vi "CAEN_HVSystem.ProcCases.vi"(0 "i ref in":refnum<vi>, 1 "selector":string, 2 "Data":T1, 3 "call cluster":T2={"Object"="", "Selector"="", "CallType"=enum."synchronous", "Async Object"="", "Async Selector"="", "Data Descriptor"="", "Data"=[], "Error #"=0, "Expire"=0}, 5 "error in (no error)":errorcluster) -> (14 "i ref out":refnum<vi>, 17 "answer cluster":T2={"Object"="", "Selector"="", "CallType"=enum."synchronous", "Async Object"="", "Async Selector"="", "Data Descriptor"="", "Data"=[], "Error #"=0, "Expire"=0}, 19 "error out":errorcluster)   [LabVIEW 2014, in "CAEN_HVSystem.lvlib"]
doc: "This method is called by a process from within the default case in the event loop. The methods of a class that are linked to events will be called from THIS method. Add your code here."
uses:
  CAEN_HVSystem.lvlib
  CS_Core/CSSystem/CoreDefs/CoreDefs.call_type.ctl
  CS_Core/BaseProcess/BaseProcess.descriptor string definition.ctl
  CS_Core/CSSystem/CoreDefs/CoreDefs.rawDataType.ctl
  CS_Core/CSApplicationBaseClasses/DeviceBase/DeviceBase.deviceState.ctl
  CSlibraries/UtilityLib/UtilityLib.valueStatus.ctl
  CS_Core/CSSystem/CoreLib/CoreLib.string 2 byte array.vi
  CS_Core/CSSystem/CoreLib/CoreLib.short 2 byte array.vi
  CS_Core/CSSystem/CoreLib/CoreLib.byte array 2 string.vi
  CS_Core/CSSystem/CoreLib/CoreLib.byte array 2 short.vi
  CS_Core/CSSystem/CoreLib/CoreLib.lvlib
  CS_Core/BaseProcess/BaseProcess.lvlib
  CS_Core/CSApplicationBaseClasses/DeviceBase/DeviceBase.lvlib
  CS_Core/CAEObj/CAEObj.lvlib
  CSlibraries-extern/DimLVEvent/LVDimInterface/LVDimInterface.lvlib
  CSlibraries/UtilityLib/UtilityLib.lvlib
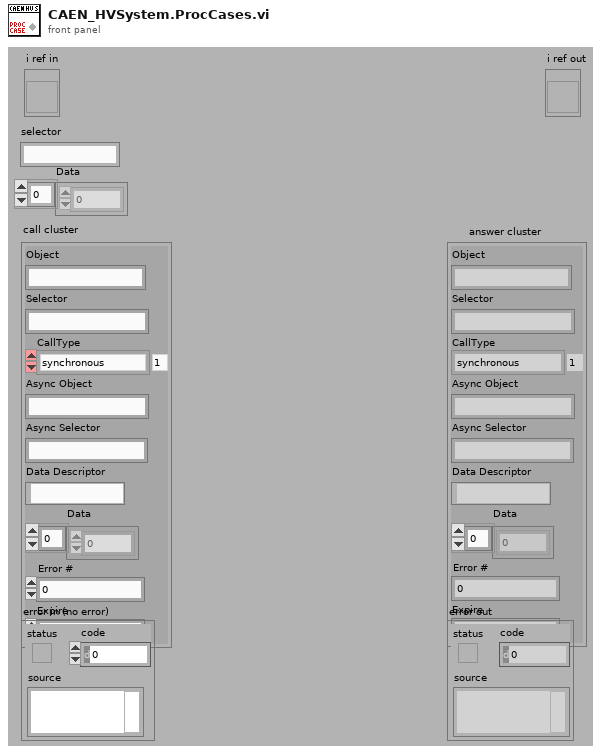
[diagram p1: front panel]
types:
  T1 = typedef "CoreDefs.rawDataType.ctl" = i8[]
  T2 = typedef "CoreDefs.call_type.ctl" = cluster{"Object":string, "Selector":string, "CallType":enum16{"simple", "synchronous", "asynchronous"}, "Async Object":string, "Async Selector":string, "Data Descriptor":T3, "Data":T1, "Error #":i32, "Expire":u32}
  T3 = typedef "BaseProcess.lvlib/BaseProcess.descriptor string definition.ctl" = string
  T4 = typedef "UtilityLib.lvlib/UtilityLib.valueStatus.ctl" = enum16{"no info available", "stand by/off", "on", "warning", "alarm/malfunction", "not implemented", "user action required", "important information", "system default", "control default", "indicator default", "button default"}
  T5 = typedef "BaseProcess.lvlib/BaseProcess.i attribute.ctl" = cluster{"EventStatus":string, "EventError":i32, "PresetEvtWatchD":i32, "PresetPdcWatchD":i32, "EventTimeout":i32, "PeriodicInterval":i32, "Interface":string[], "Address":string[], "Special":string[], "PeriodicError":i32, "PeriodicStatus":string, "SuperProc":string, "Descriptors":T6[], "CaseRef":refnum<vi>, "PdcRef":refnum<vi>, "Thread Ref":refnum<vi>, "eventErrorID":i32, "eventStatusID":i32, "periodicErrorID":i32, "periodicStatusID":i32, "pdcCtrID":i32}
  T6 = typedef "BaseProcess.lvlib/BaseProcess.descriptor definition.ctl" = cluster{"selector":string, "descriptor":T3}
  T7 = typedef "CAEN_HVSystem.lvlib/CAEN_HVSystem.i attribute.ctl" = cluster{"System Name":string, "DIM Service IDs":cluster{"Fan Status":i32}, "SymbolicName":cluster{"SymbolicName":string, "DIM Status":cluster{"no link":bool, "quality":i32, "Time Stamp":timestamp}}, "ModelName":cluster{"ModelName":string, "DIM Status":cluster{"no link":bool, "quality":i32, "Time Stamp":timestamp}}, "Slots":cluster{"Slots":i16, "DIM Status":cluster{"no link":bool, "quality":i32, "Time Stamp":timestamp}}, "Kill":cluster{"Kill":bool, "DIM Status":cluster{"no link":bool, "quality":i32, "Time Stamp":timestamp}}, "ClearAlarm":cluster{"ClearAlarm":bool, "DIM Status":cluster{"no link":bool, "quality":i32, "Time Stamp":timestamp}}, "Sessions":cluster{"Sessions":string, "DIM Status":cluster{"no link":bool, "quality":i32, "Time Stamp":timestamp}}, "SwRelease":cluster{"SwRelease":string, "DIM Status":cluster{"no link":bool, "quality":i32, "Time Stamp":timestamp}}, "GenSignCfg":cluster{"GenSignCfg":i16, "DIM Status":cluster{"no link":bool, "quality":i32, "Time Stamp":timestamp}}, "FrontPanIn":cluster{"FrontPanIn":i16, "DIM Status":cluster{"no link":bool, "quality":i32, "Time Stamp":timestamp}}, "FrontPanOut":cluster{"FrontPanOut":i16, "DIM Status":cluster{"no link":bool, "quality":i32, "Time Stamp":timestamp}}, "HvPwSM":cluster{"HvPwSM":string, "DIM Status":cluster{"no link":bool, "quality":i32, "Time Stamp":timestamp}}, "FanStat":cluster{"FanStat":string, "DIM Status":cluster{"no link":bool, "quality":i32, "Time Stamp":timestamp}}, "ClkFreq":cluster{"ClkFreq":i16, "DIM Status":cluster{"no link":bool, "quality":i32, "Time Stamp":timestamp}}, "HVClkConf":cluster{"HVClkConf":string, "DIM Status":cluster{"no link":bool, "quality":i32, "Time Stamp":timestamp}}, "CnetCrNum":cluster{"CnetCrNum":i16, "DIM Status":cluster{"no link":bool, "quality":i32, "Time Stamp":timestamp}}, "IPAddr":cluster{"IPAddr":string, "DIM Status":cluster{"no link":bool, "quality":i32, "Time Stamp":timestamp}}, "IPNetMsk":cluster{"IPNetMsk":string, "DIM Status":cluster{"no link":bool, "quality":i32, "Time Stamp":timestamp}}, "IPGw":cluster{"IPGw":string, "DIM Status":cluster{"no link":bool, "quality":i32, "Time Stamp":timestamp}}, "RS232Par":cluster{"RS232Par":string, "DIM Status":cluster{"no link":bool, "quality":i32, "Time Stamp":timestamp}}}
  T8 = typedef "DeviceBase.lvlib/DeviceBase.i attribute.ctl" = cluster{"deviceState":i32, "deviceStateID":i32, "deviceID":string, "deviceIDID":i32, "advancedGUIClass":string, "advancedGUIClassID":i32}
  T9 = typedef "DeviceBase.lvlib/DeviceBase.deviceState.ctl" = i16
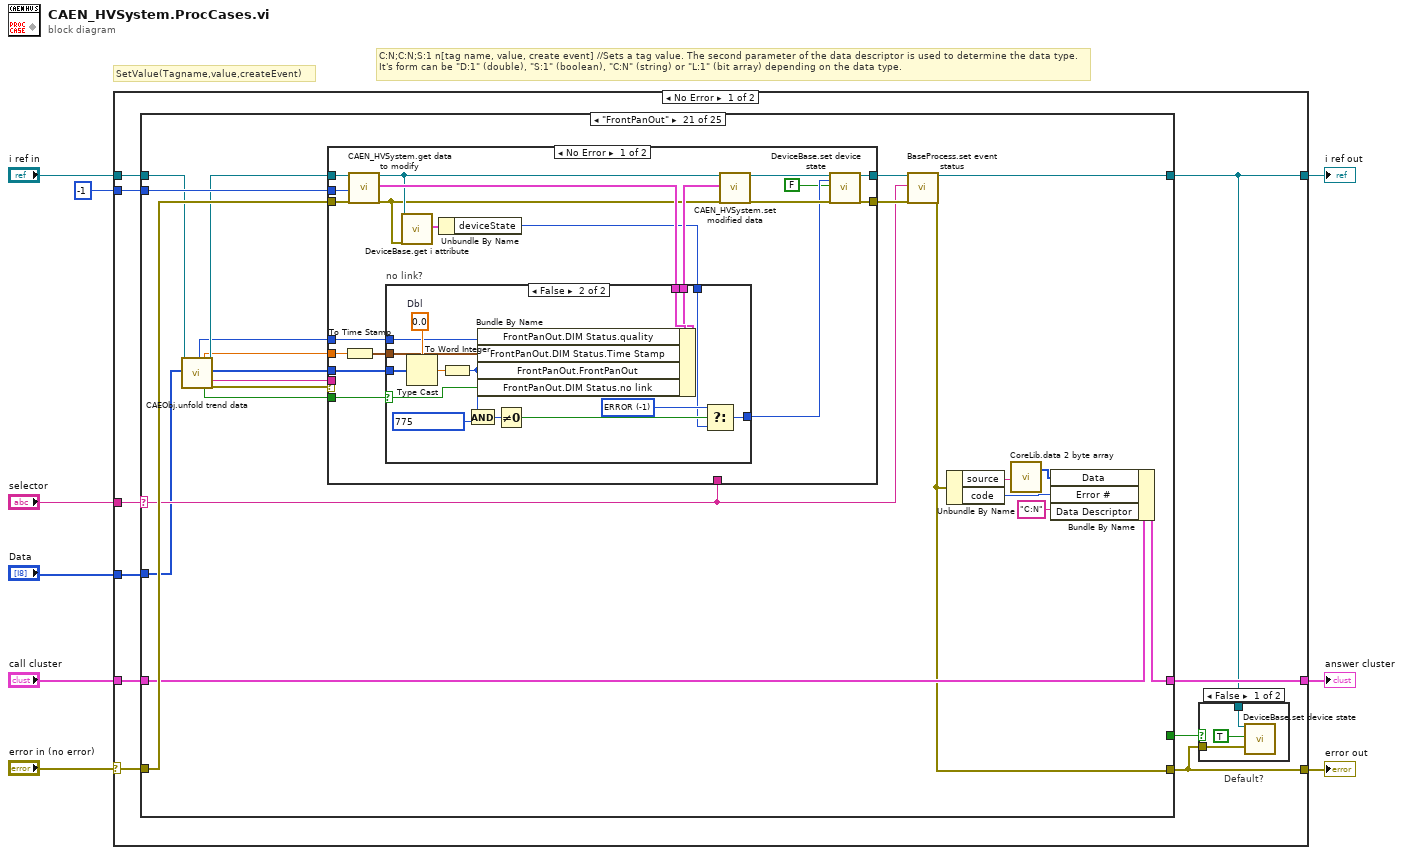
[diagram p0: block diagram]
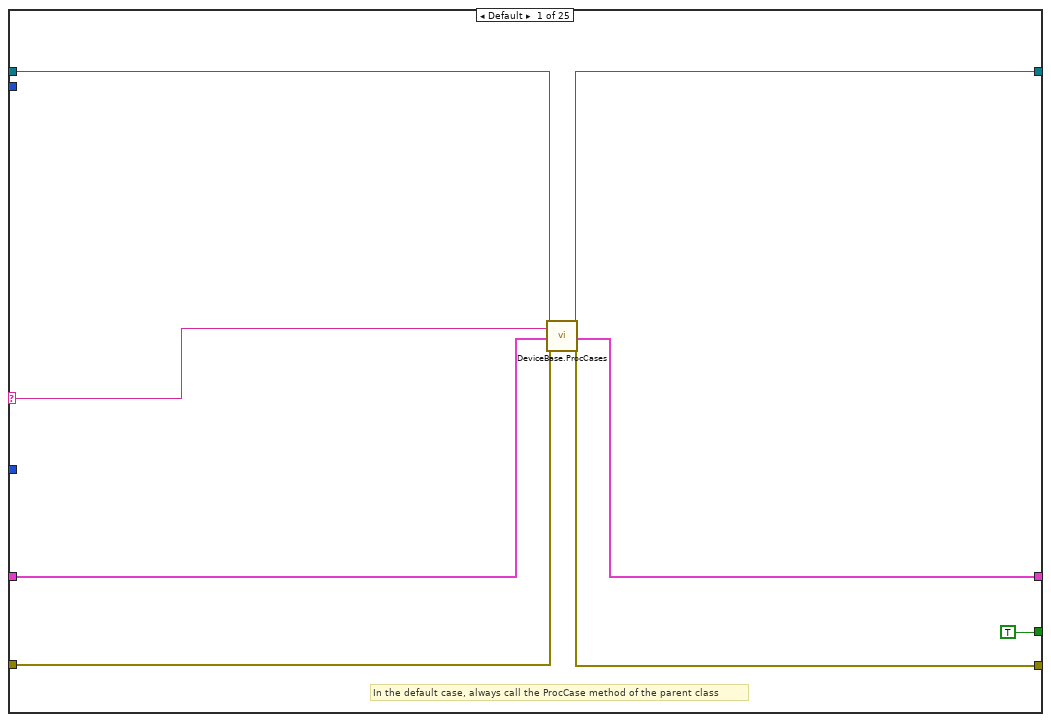
[diagram p3: hidden frame]
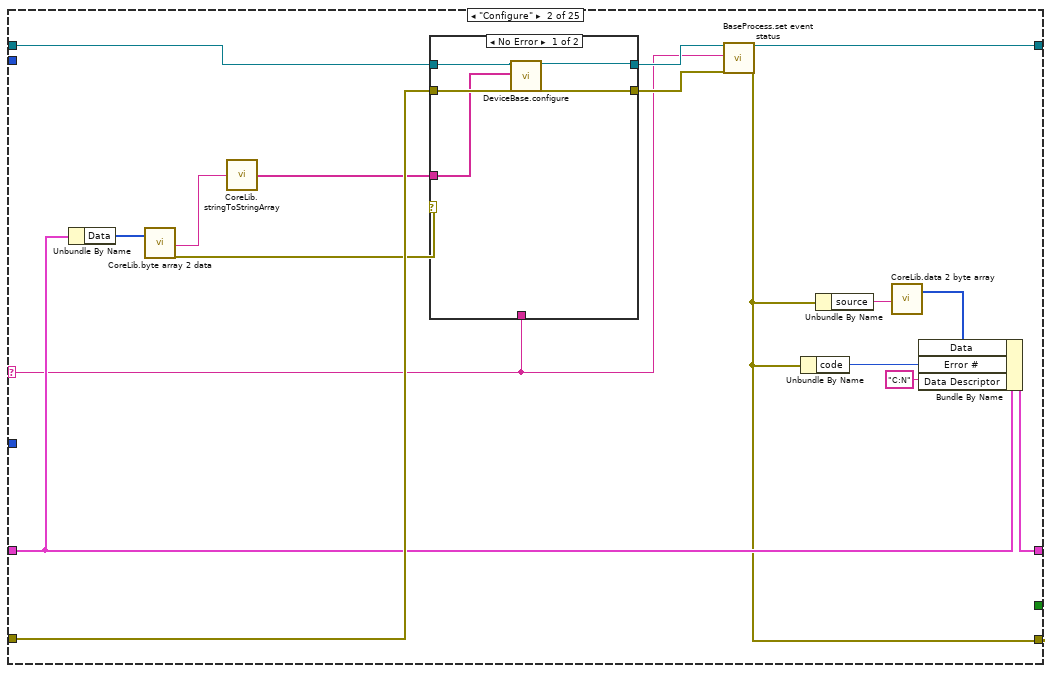
[diagram p4: hidden frame]
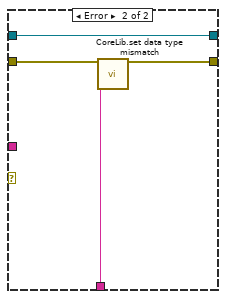
[diagram p5: hidden frame]
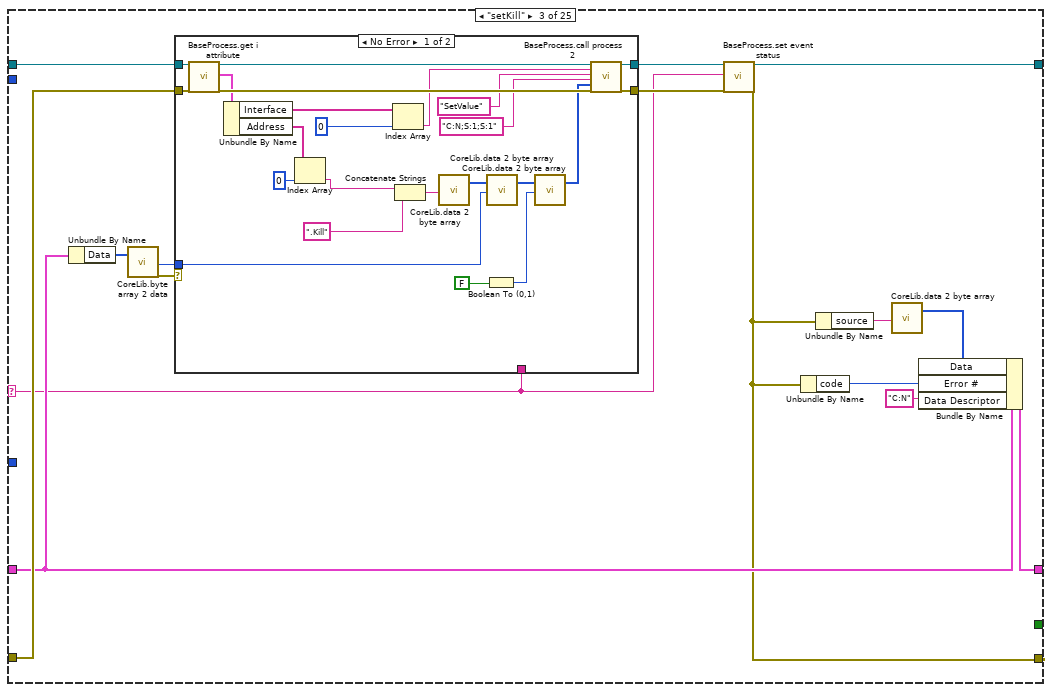
[diagram p6: hidden frame]
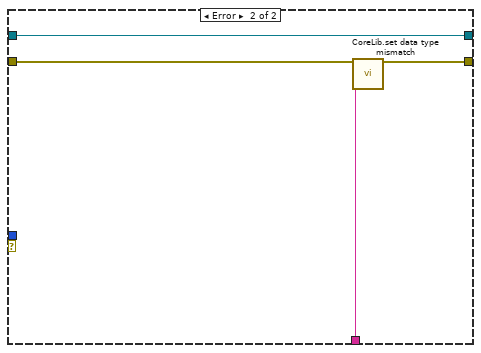
[diagram p7: hidden frame]
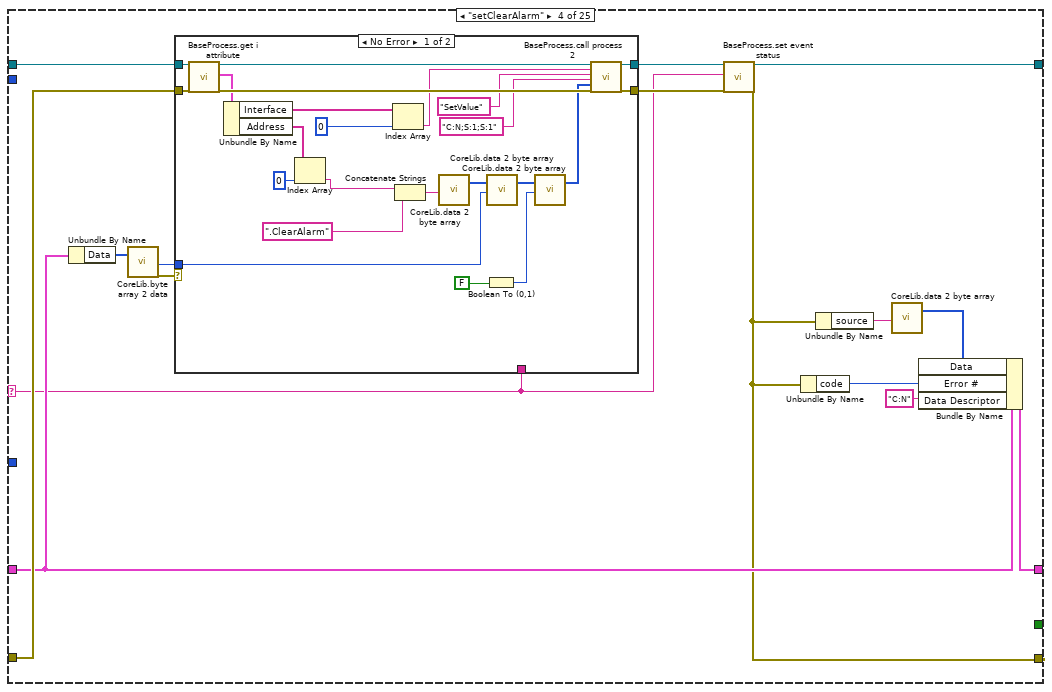
[diagram p8: hidden frame]
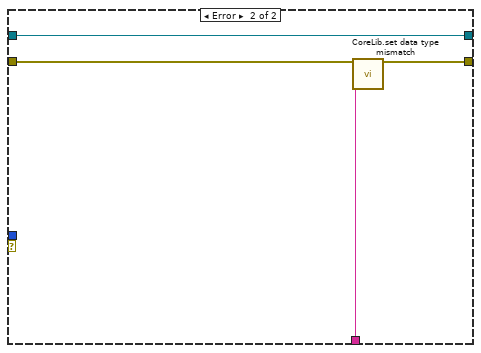
[diagram p9: hidden frame]
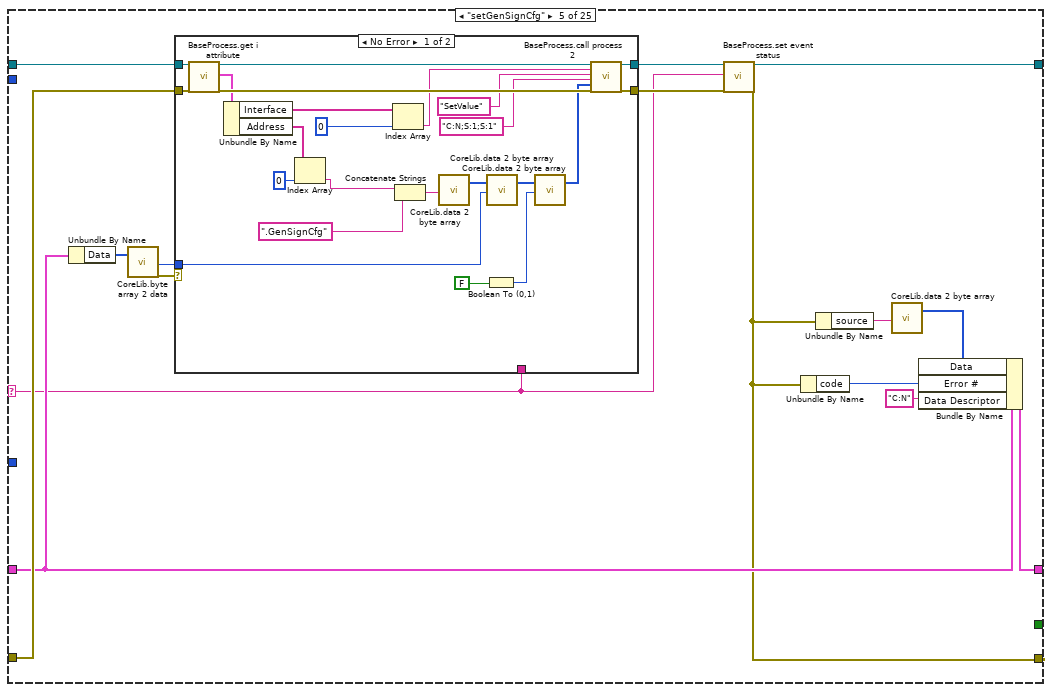
[diagram p10: hidden frame]
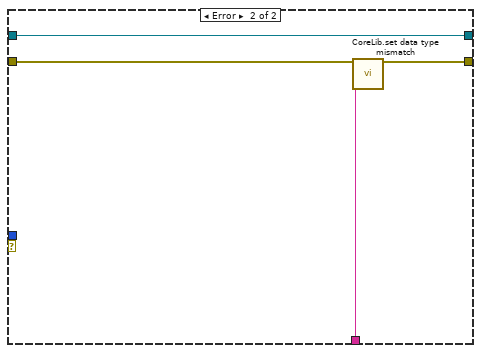
[diagram p11: hidden frame]
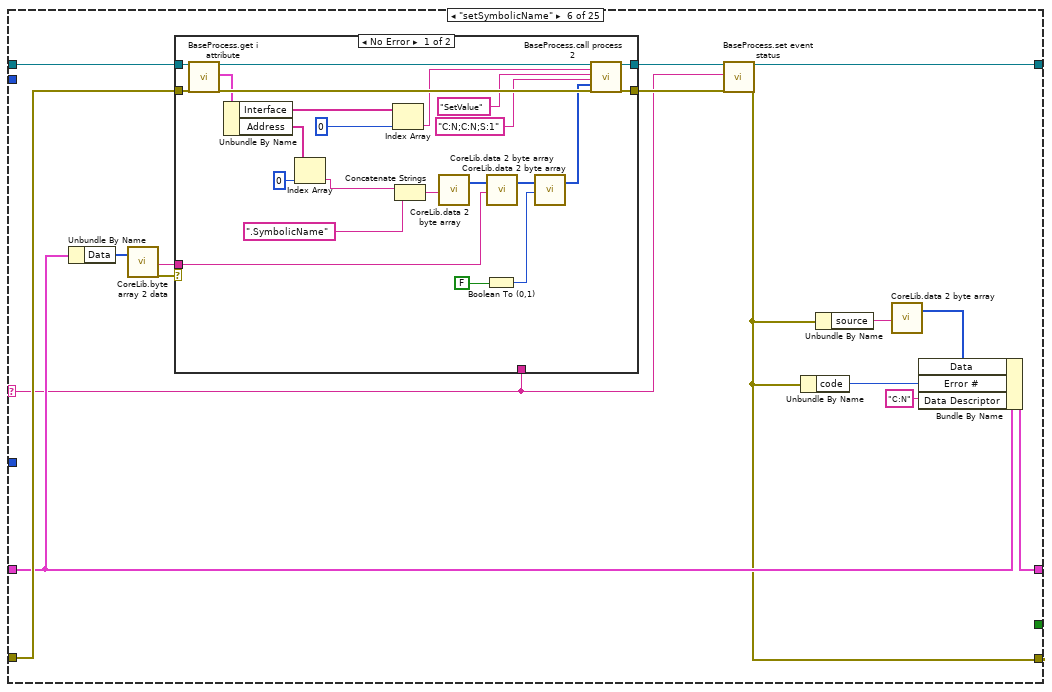
[diagram p12: hidden frame]
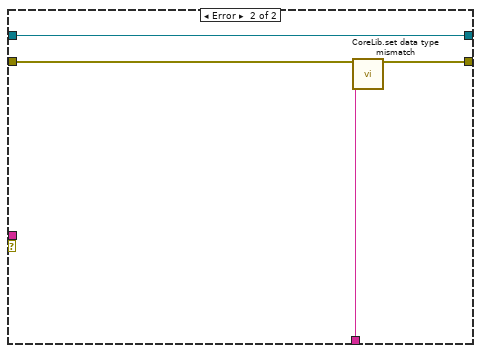
[diagram p13: hidden frame]
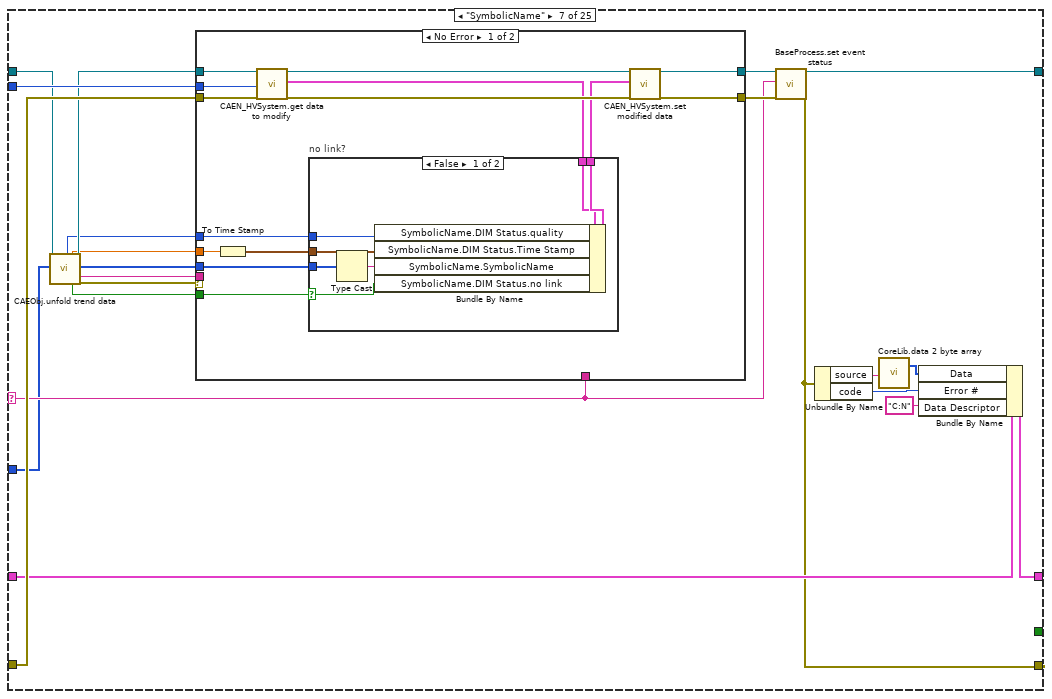
[diagram p14: hidden frame]
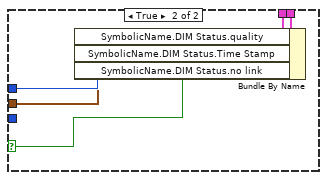
[diagram p15: hidden frame]
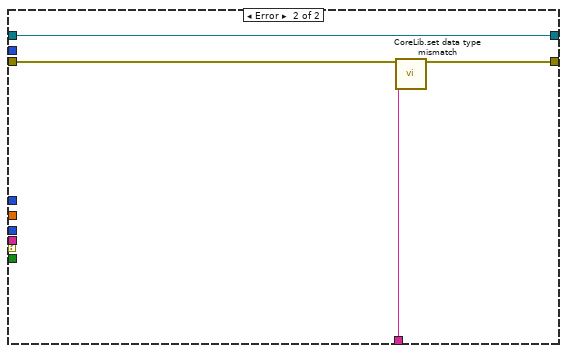
[diagram p16: hidden frame]
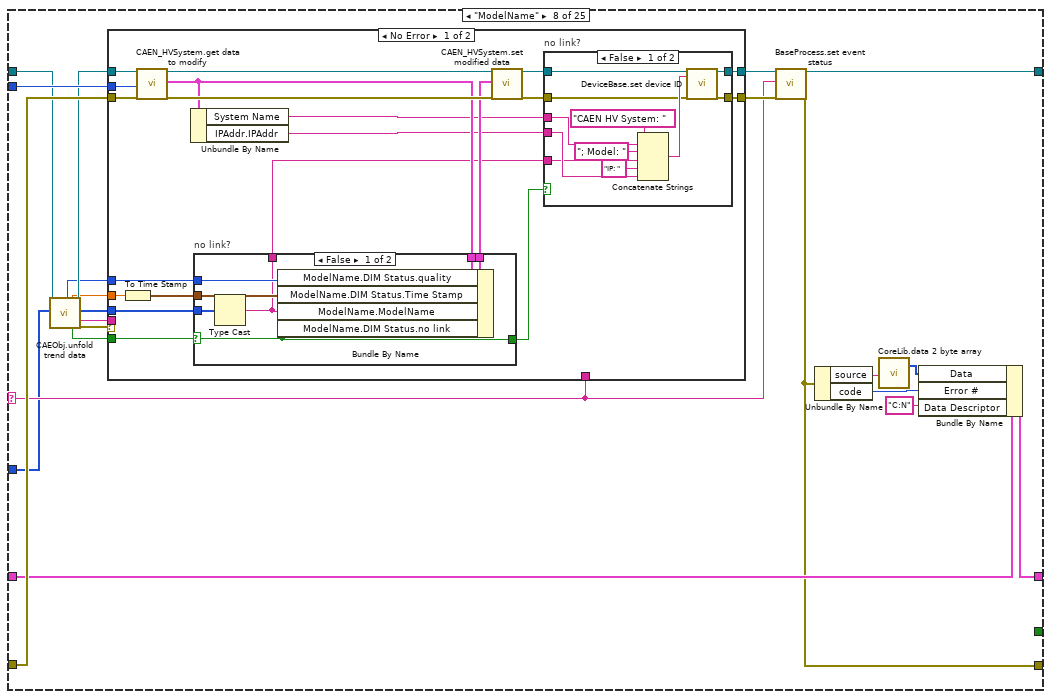
[diagram p17: hidden frame]
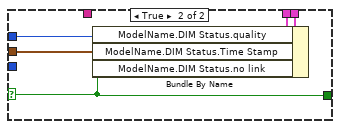
[diagram p19: hidden frame]
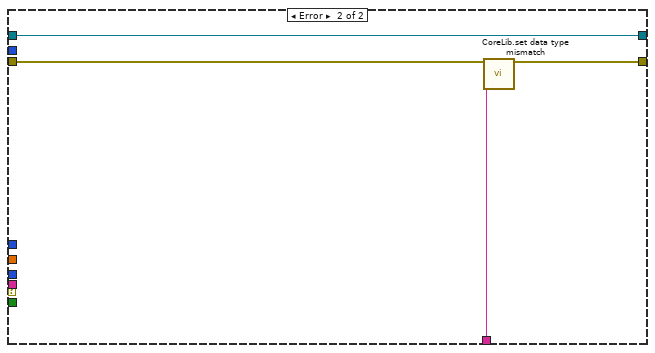
[diagram p20: hidden frame]
diagram:
  # "C:N;C:N;S:1 n[tag name, value, create event] //Sets a tag value. The second parameter of the data descriptor is used to determine the data type. It's form can be \"D:1\" (double), \"S:1\" (boolean), \"C:N\" (string) or \"L:1\" (bit array) depending on the data type."
  # "SetValue(Tagname,value,createEvent)"
  n1 = case shown="No Error" "error in (no error)" {
    selector: "error in (no error)" -> [w14 w1362]
    tunnel: "selector" -> [w19 _]
    tunnel: [w18 w1363] -> w8
    tunnel: "Data" -> [w17 _]
    tunnel: "call cluster" -> [w16 w1363]
    tunnel: "i ref in" -> [w15 w1364]
    tunnel: [w10 w1364] -> w4
    tunnel: [w12 w1362] -> w3
    tunnel: -1 ("ms timeout (10000)") -> [w13 _]
    frame No Error {
      n2 = case shown="\"FrontPanOut\"" w19 {
        selector: w19 -> [w25 w38 w62 w105 w148 w191 w241 w293 w364 w416 w468 w540 w652 w704 w775 w827 w879 w931 w985 w1039 w1093 w1159 w1213 w1267 w1321]
        tunnel: w17 -> [_ _ _ _ _ _ w237 w289 w360 w412 w464 w537 w648 w700 w771 w823 w875 w927 w981 w1035 w1089 w1155 w1209 w1263 w1317]
        tunnel: w15 -> [w24 w47 w71 w114 w157 w200 w236 w288 w359 w411 w463 w531 w647 w699 w770 w822 w874 w926 w980 w1034 w1088 w1154 w1208 w1262 w1316]
        tunnel: [w30 w37 w61 w104 w147 w190 w240 w292 w363 w415 w467 w528 w651 w703 w774 w826 w878 w930 w984 w1038 w1092 w1158 w1212 w1266 w1320] -> w10
        tunnel: w16 -> [w26 w44 w68 w111 w154 w197 w247 w299 w370 w422 w474 w546 w658 w710 w781 w833 w885 w937 w991 w1045 w1099 w1165 w1219 w1273 w1327]
        tunnel: [w27 w43 w67 w110 w153 w196 w246 w298 w369 w421 w473 w545 w657 w709 w780 w832 w884 w936 w990 w1044 w1098 w1164 w1218 w1272 w1326] -> w18
        tunnel: w14 -> [w29 w46 w70 w113 w156 w199 w249 w301 w372 w424 w476 w548 w660 w712 w783 w835 w887 w939 w993 w1047 w1101 w1167 w1221 w1275 w1329]
        tunnel: [w28 w39 w63 w106 w149 w192 w242 w294 w365 w417 w469 w541 w653 w705 w776 w828 w880 w932 w986 w1040 w1094 w1160 w1214 w1268 w1322] -> w12
        tunnel: w13 -> [_ _ _ _ _ _ w238 w290 w361 w413 w465 w538 w649 w701 w772 w824 w876 w928 w982 w1036 w1090 w1156 w1210 w1264 w1318]
        tunnel: [TRUE _ _ _ _ _ _ _ _ _ _ _ _ _ _ _ _ _ _ _ _ _ _ _ _] -> w11
        frame Default {
          # "In the default case, always call the ProcCase method of the parent class"
          n3 = call "DeviceBase.ProcCases.vi"("i ref in"=w24, "selector"=w25, "call cluster"=w26, "error in (no error)"=w29) -> ("i ref out"=w30:refnum<vi>, "answer cluster"=w27:T2, "error out"=w28:errorcluster)  [unwired: 13 in]
        }
        frame "Configure" {
          n4 = Unbundle By Name(w44) -> ("Data"=w35:T1)
          n5 = call-poly "CoreLib.byte array 2 data.vi"("byteArray"=w35) -> ("string"=w32:string, "error out"=w33:errorcluster)  [unwired: 16 in, 1 out]
          n6 = call "CoreLib.stringToStringArray.vi"("String"=w32) -> ("Array"=w31:string[])
          n7 = case shown="No Error" w33 {
            tunnel: [w49 w55] -> w41
            tunnel: w47 -> [w50 w55]
            tunnel: w46 -> [w51 w54]
            tunnel: [w51 w53] -> w40
            tunnel: w38 -> [_ w52]
            tunnel: w31 -> [w48 _]
            frame No Error {
              n8 = call "DeviceBase.configure.vi"("i ref in"=w50, "configureData"=w48) -> ("i ref out"=w49:refnum<vi>)  [unwired: 15 in, 2 out]
            }
            frame Error {
              n9 = call "CoreLib.set data type mismatch.vi"("error in (no error)"=w54, "error source"=w52) -> ("error out"=w53:errorcluster)  [unwired: 17 in]
            }
          }
          n10 = call "BaseProcess.set event status.vi"("i ref in"=w41, "EventStatus"=w38, "error in (no error)"=w40) -> ("i ref out"=w37:refnum<vi>, "error out"=w39:errorcluster)  [unwired: 14 in, 1 out]
          n11 = Unbundle By Name(w39) -> ("code"=w45:i32)
          n12 = Unbundle By Name(w39) -> ("source"=w34:string)
          n13 = call-poly "CoreLib.data 2 byte array.vi"("string"=w34) -> ("byteArray out"=w42:T1)  [unwired: 18 in]
          n14 = Bundle By Name(cluster=w44, "Data"=w42, "Error #"=w45, "Data Descriptor"="C:N") -> (w43:T2)
        }
        frame "setKill" {
          n15 = Unbundle By Name(w68) -> ("Data"=w57:T1)
          n16 = call-poly "CoreLib.byte array 2 data.vi"("byteArray"=w57) -> ("i16"=w56:i16, "error out"=w58:errorcluster)  [unwired: 16 in, 1 out]
          n17 = case shown="No Error" w58 {
            tunnel: [w94 w98] -> w65
            tunnel: w71 -> [w91 w98]
            tunnel: w70 -> [w92 w97]
            tunnel: [w93 w96] -> w64
            tunnel: w62 -> [_ w95]
            tunnel: w56 -> [w79 _]
            frame No Error {
              n18 = call "BaseProcess.get i attribute.vi"("i ref in"=w91, "error in (no error)"=w92) -> ("i ref out"=w86:refnum<vi>, "i attribute"=w89:T5, "error out"=w90:errorcluster)  [unwired: 15 in]
              n19 = Unbundle By Name(w89) -> ("Interface"=w88:string[], "Address"=w81:string[])
              n20 = Index Array(array=w81, index=0) -> (element=w74:string)
              n21 = Index Array(array=w88, index=0) -> (element=w85:string)
              n22 = Concatenate Strings(w74, ".Kill" ("string")) -> (w73:string)
              n23 = call-poly "CoreLib.data 2 byte array.vi"("string"=w73) -> ("byteArray out"=w80:T1)  [unwired: 18 in]
              n24 = Boolean To (0,1)(Boolean=FALSE) -> (0, 1=w76:i16)
              n25 = call-poly "CoreLib.data 2 byte array.vi"("byteArray"=w80, "i16"=w79) -> ("byteArray out"=w78:T1)  [unwired: 17 in]
              n26 = call-poly "CoreLib.data 2 byte array.vi"("byteArray"=w78, "i16"=w76) -> ("byteArray out"=w75:T1)  [unwired: 17 in]
              n27 = call "BaseProcess.call process 2.vi"("i ref in"=w86, "Object"=w85, "Selector"="SetValue", "Data Descriptor"="C:N;S:1;S:1", "Data"=w75, "error in (no error)"=w90) -> ("i ref out"=w94:refnum<vi>, "error out"=w93:errorcluster)  [unwired: 12 in]
            }
            frame Error {
              n28 = call "CoreLib.set data type mismatch.vi"("error in (no error)"=w97, "error source"=w95) -> ("error out"=w96:errorcluster)  [unwired: 17 in]
            }
          }
          n29 = call "BaseProcess.set event status.vi"("i ref in"=w65, "EventStatus"=w62, "error in (no error)"=w64) -> ("i ref out"=w61:refnum<vi>, "error out"=w63:errorcluster)  [unwired: 14 in, 1 out]
          n30 = Unbundle By Name(w63) -> ("code"=w69:i32)
          n31 = Unbundle By Name(w63) -> ("source"=w59:string)
          n32 = call-poly "CoreLib.data 2 byte array.vi"("string"=w59) -> ("byteArray out"=w66:T1)  [unwired: 18 in]
          n33 = Bundle By Name(cluster=w68, "Data"=w66, "Error #"=w69, "Data Descriptor"="C:N") -> (w67:T2)
        }
        frame "setClearAlarm" {
          n34 = Unbundle By Name(w111) -> ("Data"=w100:T1)
          n35 = call-poly "CoreLib.byte array 2 data.vi"("byteArray"=w100) -> ("i16"=w99:i16, "error out"=w101:errorcluster)  [unwired: 16 in, 1 out]
          n36 = case shown="No Error" w101 {
            tunnel: [w137 w141] -> w108
            tunnel: w114 -> [w134 w141]
            tunnel: w113 -> [w135 w140]
            tunnel: [w136 w139] -> w107
            tunnel: w105 -> [_ w138]
            tunnel: w99 -> [w122 _]
            frame No Error {
              n37 = call "BaseProcess.get i attribute.vi"("i ref in"=w134, "error in (no error)"=w135) -> ("i ref out"=w129:refnum<vi>, "i attribute"=w132:T5, "error out"=w133:errorcluster)  [unwired: 15 in]
              n38 = Unbundle By Name(w132) -> ("Interface"=w131:string[], "Address"=w124:string[])
              n39 = Index Array(array=w124, index=0) -> (element=w117:string)
              n40 = Index Array(array=w131, index=0) -> (element=w128:string)
              n41 = Concatenate Strings(w117, ".ClearAlarm" ("string")) -> (w116:string)
              n42 = call-poly "CoreLib.data 2 byte array.vi"("string"=w116) -> ("byteArray out"=w123:T1)  [unwired: 18 in]
              n43 = Boolean To (0,1)(Boolean=FALSE) -> (0, 1=w119:i16)
              n44 = call-poly "CoreLib.data 2 byte array.vi"("byteArray"=w123, "i16"=w122) -> ("byteArray out"=w121:T1)  [unwired: 17 in]
              n45 = call-poly "CoreLib.data 2 byte array.vi"("byteArray"=w121, "i16"=w119) -> ("byteArray out"=w118:T1)  [unwired: 17 in]
              n46 = call "BaseProcess.call process 2.vi"("i ref in"=w129, "Object"=w128, "Selector"="SetValue", "Data Descriptor"="C:N;S:1;S:1", "Data"=w118, "error in (no error)"=w133) -> ("i ref out"=w137:refnum<vi>, "error out"=w136:errorcluster)  [unwired: 12 in]
            }
            frame Error {
              n47 = call "CoreLib.set data type mismatch.vi"("error in (no error)"=w140, "error source"=w138) -> ("error out"=w139:errorcluster)  [unwired: 17 in]
            }
          }
          n48 = call "BaseProcess.set event status.vi"("i ref in"=w108, "EventStatus"=w105, "error in (no error)"=w107) -> ("i ref out"=w104:refnum<vi>, "error out"=w106:errorcluster)  [unwired: 14 in, 1 out]
          n49 = Unbundle By Name(w106) -> ("code"=w112:i32)
          n50 = Unbundle By Name(w106) -> ("source"=w102:string)
          n51 = call-poly "CoreLib.data 2 byte array.vi"("string"=w102) -> ("byteArray out"=w109:T1)  [unwired: 18 in]
          n52 = Bundle By Name(cluster=w111, "Data"=w109, "Error #"=w112, "Data Descriptor"="C:N") -> (w110:T2)
        }
        frame "setGenSignCfg" {
          n53 = Unbundle By Name(w154) -> ("Data"=w143:T1)
          n54 = call-poly "CoreLib.byte array 2 data.vi"("byteArray"=w143) -> ("i16"=w142:i16, "error out"=w144:errorcluster)  [unwired: 16 in, 1 out]
          n55 = case shown="No Error" w144 {
            tunnel: [w180 w184] -> w151
            tunnel: w157 -> [w177 w184]
            tunnel: w156 -> [w178 w183]
            tunnel: [w179 w182] -> w150
            tunnel: w148 -> [_ w181]
            tunnel: w142 -> [w165 _]
            frame No Error {
              n56 = call "BaseProcess.get i attribute.vi"("i ref in"=w177, "error in (no error)"=w178) -> ("i ref out"=w172:refnum<vi>, "i attribute"=w175:T5, "error out"=w176:errorcluster)  [unwired: 15 in]
              n57 = Unbundle By Name(w175) -> ("Interface"=w174:string[], "Address"=w167:string[])
              n58 = Index Array(array=w167, index=0) -> (element=w160:string)
              n59 = Index Array(array=w174, index=0) -> (element=w171:string)
              n60 = Concatenate Strings(w160, ".GenSignCfg" ("string")) -> (w159:string)
              n61 = call-poly "CoreLib.data 2 byte array.vi"("string"=w159) -> ("byteArray out"=w166:T1)  [unwired: 18 in]
              n62 = Boolean To (0,1)(Boolean=FALSE) -> (0, 1=w162:i16)
              n63 = call-poly "CoreLib.data 2 byte array.vi"("byteArray"=w166, "i16"=w165) -> ("byteArray out"=w164:T1)  [unwired: 17 in]
              n64 = call-poly "CoreLib.data 2 byte array.vi"("byteArray"=w164, "i16"=w162) -> ("byteArray out"=w161:T1)  [unwired: 17 in]
              n65 = call "BaseProcess.call process 2.vi"("i ref in"=w172, "Object"=w171, "Selector"="SetValue", "Data Descriptor"="C:N;S:1;S:1", "Data"=w161, "error in (no error)"=w176) -> ("i ref out"=w180:refnum<vi>, "error out"=w179:errorcluster)  [unwired: 12 in]
            }
            frame Error {
              n66 = call "CoreLib.set data type mismatch.vi"("error in (no error)"=w183, "error source"=w181) -> ("error out"=w182:errorcluster)  [unwired: 17 in]
            }
          }
          n67 = call "BaseProcess.set event status.vi"("i ref in"=w151, "EventStatus"=w148, "error in (no error)"=w150) -> ("i ref out"=w147:refnum<vi>, "error out"=w149:errorcluster)  [unwired: 14 in, 1 out]
          n68 = Unbundle By Name(w149) -> ("code"=w155:i32)
          n69 = Unbundle By Name(w149) -> ("source"=w145:string)
          n70 = call-poly "CoreLib.data 2 byte array.vi"("string"=w145) -> ("byteArray out"=w152:T1)  [unwired: 18 in]
          n71 = Bundle By Name(cluster=w154, "Data"=w152, "Error #"=w155, "Data Descriptor"="C:N") -> (w153:T2)
        }
        frame "setSymbolicName" {
          n72 = Unbundle By Name(w197) -> ("Data"=w186:T1)
          n73 = call-poly "CoreLib.byte array 2 data.vi"("byteArray"=w186) -> ("string"=w185:string, "error out"=w187:errorcluster)  [unwired: 16 in, 1 out]
          n74 = case shown="No Error" w187 {
            tunnel: [w223 w227] -> w194
            tunnel: w200 -> [w220 w227]
            tunnel: w199 -> [w221 w226]
            tunnel: [w222 w225] -> w193
            tunnel: w191 -> [_ w224]
            tunnel: w185 -> [w208 _]
            frame No Error {
              n75 = call "BaseProcess.get i attribute.vi"("i ref in"=w220, "error in (no error)"=w221) -> ("i ref out"=w215:refnum<vi>, "i attribute"=w218:T5, "error out"=w219:errorcluster)  [unwired: 15 in]
              n76 = Unbundle By Name(w218) -> ("Interface"=w217:string[], "Address"=w210:string[])
              n77 = Index Array(array=w210, index=0) -> (element=w203:string)
              n78 = Index Array(array=w217, index=0) -> (element=w214:string)
              n79 = Concatenate Strings(w203, ".SymbolicName" ("string")) -> (w202:string)
              n80 = call-poly "CoreLib.data 2 byte array.vi"("string"=w202) -> ("byteArray out"=w209:T1)  [unwired: 18 in]
              n81 = Boolean To (0,1)(Boolean=FALSE) -> (0, 1=w205:i16)
              n82 = call-poly "CoreLib.data 2 byte array.vi"("byteArray"=w209, "string"=w208) -> ("byteArray out"=w207:T1)  [unwired: 17 in]
              n83 = call-poly "CoreLib.data 2 byte array.vi"("byteArray"=w207, "i16"=w205) -> ("byteArray out"=w204:T1)  [unwired: 17 in]
              n84 = call "BaseProcess.call process 2.vi"("i ref in"=w215, "Object"=w214, "Selector"="SetValue", "Data Descriptor"="C:N;C:N;S:1", "Data"=w204, "error in (no error)"=w219) -> ("i ref out"=w223:refnum<vi>, "error out"=w222:errorcluster)  [unwired: 12 in]
            }
            frame Error {
              n85 = call "CoreLib.set data type mismatch.vi"("error in (no error)"=w226, "error source"=w224) -> ("error out"=w225:errorcluster)  [unwired: 17 in]
            }
          }
          n86 = call "BaseProcess.set event status.vi"("i ref in"=w194, "EventStatus"=w191, "error in (no error)"=w193) -> ("i ref out"=w190:refnum<vi>, "error out"=w192:errorcluster)  [unwired: 14 in, 1 out]
          n87 = Unbundle By Name(w192) -> ("code"=w198:i32)
          n88 = Unbundle By Name(w192) -> ("source"=w188:string)
          n89 = call-poly "CoreLib.data 2 byte array.vi"("string"=w188) -> ("byteArray out"=w195:T1)  [unwired: 18 in]
          n90 = Bundle By Name(cluster=w197, "Data"=w195, "Error #"=w198, "Data Descriptor"="C:N") -> (w196:T2)
        }
        frame "SymbolicName" {
          n91 = call "CAEObj.unfold trend data.vi"("i ref in"=w236, "raw trend data"=w237) -> ("quality"=w230:i32, "timeStamp"=w229:dbl, "no link"=w231:bool, "i ref out"=w235:refnum<vi>, "data"=w234:i8[], "typeDescriptor"=w232:string, "error out"=w228:errorcluster)  [unwired: 9 in, 2 out]
          n92 = case shown="No Error" w228 {
            tunnel: [w255 w279] -> w244
            tunnel: w235 -> [w263 w279]
            tunnel: w249 -> [w262 w278]
            tunnel: [w254 w277] -> w243
            tunnel: w241 -> [_ w276]
            tunnel: w238 -> [w261 _]
            tunnel: w234 -> [w257 _]
            tunnel: w232 -> [_ _]
            tunnel: w231 -> [w250 _]
            tunnel: w230 -> [w253 _]
            tunnel: w229 -> [w252 _]
            frame No Error {
              n93 = To Time Stamp(1:w252) -> (0:w251:timestamp)
              n94 = call "CAEN_HVSystem.get data to modify.vi"("i ref in"=w263, "ms timeout (10000)"=w261, "error in (no error)"=w262) -> ("i ref out"=w260:refnum<vi>, "i attribute"=w256:T7, "error out"=w259:errorcluster)  [unwired: 13 in, 1 out]
              n95 = case "no link?" shown="False" w250 {
                selector: w250 -> [w264 w271]
                tunnel: [w270 w275] -> w258
                tunnel: w257 -> [w269 _]
                tunnel: w256 -> [w267 w274]
                tunnel: w253 -> [w266 w273]
                tunnel: w251 -> [w265 w272]
                frame False {
                  n96 = Type Cast(x=w269) -> (*(type *) &x=w268:string)  [unwired: 1 in]
                  n97 = Bundle By Name(cluster=w267, "SymbolicName.DIM Status.quality"=w266, "SymbolicName.DIM Status.Time Stamp"=w265, "SymbolicName.SymbolicName"=w268, "SymbolicName.DIM Status.no link"=w264) -> (w270:T7)
                }
                frame True {
                  n98 = Bundle By Name(cluster=w274, "SymbolicName.DIM Status.quality"=w273, "SymbolicName.DIM Status.Time Stamp"=w272, "SymbolicName.DIM Status.no link"=w271) -> (w275:T7)
                }
              }
              n99 = call "CAEN_HVSystem.set modified data.vi"("i ref in"=w260, "i attribute"=w258, "error in (no error)"=w259) -> ("i ref out"=w255:refnum<vi>, "error out"=w254:errorcluster)  [unwired: 15 in]
            }
            frame Error {
              n100 = call "CoreLib.set data type mismatch.vi"("error in (no error)"=w278, "error source"=w276) -> ("error out"=w277:errorcluster)  [unwired: 17 in]
            }
          }
          n101 = call "BaseProcess.set event status.vi"("i ref in"=w244, "EventStatus"=w241, "error in (no error)"=w243) -> ("i ref out"=w240:refnum<vi>, "error out"=w242:errorcluster)  [unwired: 14 in, 1 out]
          n102 = Unbundle By Name(w242) -> ("source"=w233:string, "code"=w248:i32)
          n103 = call-poly "CoreLib.data 2 byte array.vi"("string"=w233) -> ("byteArray out"=w245:T1)  [unwired: 18 in]
          n104 = Bundle By Name(cluster=w247, "Data"=w245, "Error #"=w248, "Data Descriptor"="C:N") -> (w246:T2)
        }
        frame "ModelName" {
          n105 = call "CAEObj.unfold trend data.vi"("i ref in"=w288, "raw trend data"=w289) -> ("quality"=w282:i32, "timeStamp"=w281:dbl, "no link"=w280:bool, "i ref out"=w287:refnum<vi>, "data"=w286:i8[], "typeDescriptor"=w284:string, "error out"=w283:errorcluster)  [unwired: 9 in, 2 out]
          n106 = case shown="No Error" w283 {
            tunnel: [w314 w350] -> w296
            tunnel: w287 -> [w321 w350]
            tunnel: w301 -> [w320 w349]
            tunnel: [w313 w348] -> w295
            tunnel: w293 -> [_ w347]
            tunnel: w290 -> [w319 _]
            tunnel: w286 -> [w315 _]
            tunnel: w284 -> [_ _]
            tunnel: w282 -> [w307 _]
            tunnel: w281 -> [w306 _]
            tunnel: w280 -> [w303 _]
            frame No Error {
              n107 = To Time Stamp(1:w306) -> (0:w305:timestamp)
              n108 = call "CAEN_HVSystem.get data to modify.vi"("i ref in"=w321, "ms timeout (10000)"=w319, "error in (no error)"=w320) -> ("i ref out"=w318:refnum<vi>, "i attribute"=w310:T7, "error out"=w317:errorcluster)  [unwired: 13 in, 1 out]
              n109 = Unbundle By Name(w310) -> ("System Name"=w309:string, "IPAddr.IPAddr"=w308:string)
              n110 = case "no link?" shown="False" w303 {
                selector: w303 -> [w335 w342]
                tunnel: [w341 w346] -> w316
                tunnel: w315 -> [w340 _]
                tunnel: w310 -> [w339 w345]
                tunnel: w307 -> [w338 w344]
                tunnel: w305 -> [w337 w343]
                tunnel: [w336 _] -> w304
                tunnel: [w335 w342] -> w302
                frame False {
                  n111 = Type Cast(x=w340) -> (*(type *) &x=w336:string)  [unwired: 1 in]
                  n112 = Bundle By Name(cluster=w339, "ModelName.DIM Status.quality"=w338, "ModelName.DIM Status.Time Stamp"=w337, "ModelName.ModelName"=w336, "ModelName.DIM Status.no link"=w335) -> (w341:T7)
                }
                frame True {
                  n113 = Bundle By Name(cluster=w345, "ModelName.DIM Status.quality"=w344, "ModelName.DIM Status.Time Stamp"=w343, "ModelName.DIM Status.no link"=w342) -> (w346:T7)
                }
              }
              n114 = call "CAEN_HVSystem.set modified data.vi"("i ref in"=w318, "i attribute"=w316, "error in (no error)"=w317) -> ("i ref out"=w311:refnum<vi>, "error out"=w312:errorcluster)  [unwired: 15 in]
              n115 = case "no link?" shown="False" w302 {
                tunnel: [w328 w334] -> w314
                tunnel: [w327 w333] -> w313
                tunnel: w312 -> [w326 w333]
                tunnel: w311 -> [w325 w334]
                tunnel: w309 -> [w324 _]
                tunnel: w308 -> [w323 _]
                tunnel: w304 -> [w322 _]
                frame False {
                  n116 = Concatenate Strings("CAEN HV System: " ("string"), w324, "; Model: " ("string"), w322, "IP: " ("string"), w323) -> (w332:string)
                  n117 = call "DeviceBase.set device ID.vi"("i ref in"=w325, "deviceID"=w332, "error in (no error)"=w326) -> ("i ref out"=w328:refnum<vi>, "error out"=w327:errorcluster)  [unwired: 14 in, 1 out]
                }
                frame True {
                }
              }
            }
            frame Error {
              n118 = call "CoreLib.set data type mismatch.vi"("error in (no error)"=w349, "error source"=w347) -> ("error out"=w348:errorcluster)  [unwired: 17 in]
            }
          }
          n119 = call "BaseProcess.set event status.vi"("i ref in"=w296, "EventStatus"=w293, "error in (no error)"=w295) -> ("i ref out"=w292:refnum<vi>, "error out"=w294:errorcluster)  [unwired: 14 in, 1 out]
          n120 = Unbundle By Name(w294) -> ("source"=w285:string, "code"=w300:i32)
          n121 = call-poly "CoreLib.data 2 byte array.vi"("string"=w285) -> ("byteArray out"=w297:T1)  [unwired: 18 in]
          n122 = Bundle By Name(cluster=w299, "Data"=w297, "Error #"=w300, "Data Descriptor"="C:N") -> (w298:T2)
        }
        frame "Sessions" {
          n123 = call "CAEObj.unfold trend data.vi"("i ref in"=w359, "raw trend data"=w360) -> ("quality"=w352:i32, "timeStamp"=w351:dbl, "no link"=w353:bool, "i ref out"=w358:refnum<vi>, "data"=w357:i8[], "typeDescriptor"=w355:string, "error out"=w354:errorcluster)  [unwired: 9 in, 2 out]
          n124 = case shown="No Error" w354 {
            tunnel: [w379 w402] -> w367
            tunnel: w358 -> [w386 w402]
            tunnel: w372 -> [w385 w401]
            tunnel: [w380 w400] -> w366
            tunnel: w364 -> [_ w399]
            tunnel: w361 -> [w384 _]
            tunnel: w357 -> [w377 _]
            tunnel: w355 -> [_ _]
            tunnel: w353 -> [w373 _]
            tunnel: w352 -> [w376 _]
            tunnel: w351 -> [w375 _]
            frame No Error {
              n125 = call "CAEN_HVSystem.get data to modify.vi"("i ref in"=w386, "ms timeout (10000)"=w384, "error in (no error)"=w385) -> ("i ref out"=w382:refnum<vi>, "i attribute"=w383:T7, "error out"=w381:errorcluster)  [unwired: 13 in, 1 out]
              n126 = To Time Stamp(1:w375) -> (0:w374:timestamp)
              n127 = case "no link?" shown="False" w373 {
                selector: w373 -> [w387 w392]
                tunnel: w383 -> [w391 w398]
                tunnel: [w390 w397] -> w378
                tunnel: w377 -> [_ w396]
                tunnel: w376 -> [w389 w394]
                tunnel: w374 -> [w388 w393]
                frame True {
                  n128 = Bundle By Name(cluster=w391, "Sessions.DIM Status.quality"=w389, "Sessions.DIM Status.Time Stamp"=w388, "Sessions.DIM Status.no link"=w387) -> (w390:T7)
                }
                frame False {
                  n129 = Type Cast(x=w396) -> (*(type *) &x=w395:string)  [unwired: 1 in]
                  n130 = Bundle By Name(cluster=w398, "Sessions.DIM Status.quality"=w394, "Sessions.DIM Status.Time Stamp"=w393, "Sessions.Sessions"=w395, "Sessions.DIM Status.no link"=w392) -> (w397:T7)
                }
              }
              n131 = call "CAEN_HVSystem.set modified data.vi"("i ref in"=w382, "i attribute"=w378, "error in (no error)"=w381) -> ("i ref out"=w379:refnum<vi>, "error out"=w380:errorcluster)  [unwired: 15 in]
            }
            frame Error {
              n132 = call "CoreLib.set data type mismatch.vi"("error in (no error)"=w401, "error source"=w399) -> ("error out"=w400:errorcluster)  [unwired: 17 in]
            }
          }
          n133 = call "BaseProcess.set event status.vi"("i ref in"=w367, "EventStatus"=w364, "error in (no error)"=w366) -> ("i ref out"=w363:refnum<vi>, "error out"=w365:errorcluster)  [unwired: 14 in, 1 out]
          n134 = Unbundle By Name(w365) -> ("source"=w356:string, "code"=w371:i32)
          n135 = call-poly "CoreLib.data 2 byte array.vi"("string"=w356) -> ("byteArray out"=w368:T1)  [unwired: 18 in]
          n136 = Bundle By Name(cluster=w370, "Data"=w368, "Error #"=w371, "Data Descriptor"="C:N") -> (w369:T2)
        }
        frame "SwRelease" {
          n137 = call "CAEObj.unfold trend data.vi"("i ref in"=w411, "raw trend data"=w412) -> ("quality"=w403:i32, "timeStamp"=w404:dbl, "no link"=w405:bool, "i ref out"=w410:refnum<vi>, "data"=w409:i8[], "typeDescriptor"=w407:string, "error out"=w406:errorcluster)  [unwired: 9 in, 2 out]
          n138 = case shown="No Error" w406 {
            tunnel: [w431 w454] -> w419
            tunnel: w410 -> [w438 w454]
            tunnel: w424 -> [w437 w453]
            tunnel: [w432 w452] -> w418
            tunnel: w416 -> [_ w451]
            tunnel: w413 -> [w436 _]
            tunnel: w409 -> [w429 _]
            tunnel: w407 -> [_ _]
            tunnel: w405 -> [w425 _]
            tunnel: w404 -> [w428 _]
            tunnel: w403 -> [w426 _]
            frame No Error {
              n139 = call "CAEN_HVSystem.get data to modify.vi"("i ref in"=w438, "ms timeout (10000)"=w436, "error in (no error)"=w437) -> ("i ref out"=w434:refnum<vi>, "i attribute"=w435:T7, "error out"=w433:errorcluster)  [unwired: 13 in, 1 out]
              n140 = To Time Stamp(1:w428) -> (0:w427:timestamp)
              n141 = case "no link?" shown="False" w425 {
                selector: w425 -> [w439 w444]
                tunnel: w435 -> [w443 w450]
                tunnel: [w442 w449] -> w430
                tunnel: w429 -> [_ w448]
                tunnel: w427 -> [w441 w446]
                tunnel: w426 -> [w440 w445]
                frame True {
                  n142 = Bundle By Name(cluster=w443, "SwRelease.DIM Status.quality"=w440, "SwRelease.DIM Status.Time Stamp"=w441, "SwRelease.DIM Status.no link"=w439) -> (w442:T7)
                }
                frame False {
                  n143 = Type Cast(x=w448) -> (*(type *) &x=w447:string)  [unwired: 1 in]
                  n144 = Bundle By Name(cluster=w450, "SwRelease.DIM Status.quality"=w445, "SwRelease.DIM Status.Time Stamp"=w446, "SwRelease.SwRelease"=w447, "SwRelease.DIM Status.no link"=w444) -> (w449:T7)
                }
              }
              n145 = call "CAEN_HVSystem.set modified data.vi"("i ref in"=w434, "i attribute"=w430, "error in (no error)"=w433) -> ("i ref out"=w431:refnum<vi>, "error out"=w432:errorcluster)  [unwired: 15 in]
            }
            frame Error {
              n146 = call "CoreLib.set data type mismatch.vi"("error in (no error)"=w453, "error source"=w451) -> ("error out"=w452:errorcluster)  [unwired: 17 in]
            }
          }
          n147 = call "BaseProcess.set event status.vi"("i ref in"=w419, "EventStatus"=w416, "error in (no error)"=w418) -> ("i ref out"=w415:refnum<vi>, "error out"=w417:errorcluster)  [unwired: 14 in, 1 out]
          n148 = Unbundle By Name(w417) -> ("source"=w408:string, "code"=w423:i32)
          n149 = call-poly "CoreLib.data 2 byte array.vi"("string"=w408) -> ("byteArray out"=w420:T1)  [unwired: 18 in]
          n150 = Bundle By Name(cluster=w422, "Data"=w420, "Error #"=w423, "Data Descriptor"="C:N") -> (w421:T2)
        }
        frame "HvPwSM" {
          n151 = call "CAEObj.unfold trend data.vi"("i ref in"=w463, "raw trend data"=w464) -> ("quality"=w457:i32, "timeStamp"=w458:dbl, "no link"=w455:bool, "i ref out"=w462:refnum<vi>, "data"=w461:i8[], "typeDescriptor"=w459:string, "error out"=w456:errorcluster)  [unwired: 9 in, 2 out]
          n152 = case shown="No Error" w456 {
            tunnel: [w485 w519] -> w471
            tunnel: w462 -> [w496 w519]
            tunnel: w476 -> [w495 w518]
            tunnel: [w484 w517] -> w470
            tunnel: w468 -> [_ w516]
            tunnel: w465 -> [w494 _]
            tunnel: w461 -> [w491 _]
            tunnel: w459 -> [_ _]
            tunnel: w458 -> [w490 _]
            tunnel: w457 -> [w489 _]
            tunnel: w455 -> [w487 _]
            frame No Error {
              n153 = To Time Stamp(1:w490) -> (0:w488:timestamp)
              n154 = call "CAEN_HVSystem.get data to modify.vi"("i ref in"=w496, "ms timeout (10000)"=w494, "error in (no error)"=w495) -> ("i ref out"=w481:refnum<vi>, "i attribute"=w493:T7, "error out"=w480:errorcluster)  [unwired: 13 in, 1 out]
              n155 = call "DeviceBase.get i attribute.vi"("i ref in"=w481, "error in (no error)"=w480) -> ("i attribute"=w482:T8)  [unwired: 15 in, 2 out]
              n156 = Unbundle By Name(w482) -> ("deviceState"=w479:i32)
              n157 = case "no link?" shown="False" w487 {
                selector: w487 -> [w498 w510]
                tunnel: w493 -> [w502 w515]
                tunnel: [w501 w514] -> w492
                tunnel: w491 -> [_ w513]
                tunnel: w489 -> [w500 w512]
                tunnel: w488 -> [w499 w511]
                tunnel: w479 -> [w497 w504]
                tunnel: [w497 w503] -> w478
                frame True {
                  n158 = Bundle By Name(cluster=w502, "HvPwSM.DIM Status.quality"=w500, "HvPwSM.DIM Status.Time Stamp"=w499, "HvPwSM.DIM Status.no link"=w498) -> (w501:T7)
                }
                frame False {
                  w507 = T9 -1 items=["ERROR"=-1, "OK"=0, "NOT_OK"=1] ("deviceState")
                  n159 = Type Cast(x=w513) -> (*(type *) &x=w509:string)  [unwired: 1 in]
                  n160 = Bundle By Name(cluster=w515, "HvPwSM.DIM Status.quality"=w512, "HvPwSM.DIM Status.Time Stamp"=w511, "HvPwSM.HvPwSM"=w509, "HvPwSM.DIM Status.no link"=w510) -> (w514:T7)
                  n161 = Match Pattern(string=w509, regular expression="-1") -> (offset past match=w506:i32)  [unwired: 1 in, 3 out]
                  n162 = Less Than 0?(x=w506) -> (x < 0?=w505:bool)
                  n163 = Select(t=w507, s=w505, f=w504) -> (s? t:f=w503:i32)
                }
              }
              n164 = call "CAEN_HVSystem.set modified data.vi"("i ref in"=w481, "i attribute"=w492, "error in (no error)"=w480) -> ("i ref out"=w486:refnum<vi>, "error out"=w483:errorcluster)  [unwired: 15 in]
              n165 = call "DeviceBase.set device state.vi"("i ref in"=w486, "deviceState"=w478, "implicit"=FALSE, "error in (no error)"=w483) -> ("i ref out"=w485:refnum<vi>, "error out"=w484:errorcluster)  [unwired: 13 in, 1 out]
            }
            frame Error {
              n166 = call "CoreLib.set data type mismatch.vi"("error in (no error)"=w518, "error source"=w516) -> ("error out"=w517:errorcluster)  [unwired: 17 in]
            }
          }
          n167 = call "BaseProcess.set event status.vi"("i ref in"=w471, "EventStatus"=w468, "error in (no error)"=w470) -> ("i ref out"=w467:refnum<vi>, "error out"=w469:errorcluster)  [unwired: 14 in, 1 out]
          n168 = Unbundle By Name(w469) -> ("source"=w460:string, "code"=w475:i32)
          n169 = call-poly "CoreLib.data 2 byte array.vi"("string"=w460) -> ("byteArray out"=w472:T1)  [unwired: 18 in]
          n170 = Bundle By Name(cluster=w474, "Data"=w472, "Error #"=w475, "Data Descriptor"="C:N") -> (w473:T2)
        }
        frame "FanStat" {
          n171 = call "CAEObj.unfold trend data.vi"("i ref in"=w531, "raw trend data"=w537) -> ("quality"=w522:i32, "timeStamp"=w524:dbl, "no link"=w523:bool, "i ref out"=w532:refnum<vi>, "data"=w536:i8[], "typeDescriptor"=w534:string, "error out"=w526:errorcluster)  [unwired: 9 in, 2 out]
          n172 = case shown="No Error" w526 {
            tunnel: [w564 w638] -> w543
            tunnel: w532 -> [w570 w638]
            tunnel: w548 -> [w569 w637]
            tunnel: [w565 w636] -> w542
            tunnel: w540 -> [_ w635]
            tunnel: w538 -> [w568 _]
            tunnel: w536 -> [w562 _]
            tunnel: w534 -> [_ _]
            tunnel: [w559 UtilityLib.valueStatus."no info available" ("valueStatus")] -> w521
            tunnel: [w558 _] -> w520
            tunnel: w524 -> [w556 _]
            tunnel: w523 -> [w551 _]
            tunnel: w522 -> [w554 _]
            frame No Error {
              n173 = To Time Stamp(1:w556) -> (0:w555:timestamp)
              n174 = call "CAEN_HVSystem.get data to modify.vi"("i ref in"=w570, "ms timeout (10000)"=w568, "error in (no error)"=w569) -> ("i ref out"=w567:refnum<vi>, "i attribute"=w561:T7, "error out"=w566:errorcluster)  [unwired: 13 in, 1 out]
              n175 = Unbundle By Name(w561) -> ("FanStat.FanStat"=w553:string, "ModelName.ModelName"=w560:string)
              n176 = Not Equal?(x=w560, y="SY2527") -> (x != y?=w552:bool)
              n177 = case "no link?" shown="False" w551 {
                selector: w551 -> [w573 w628]
                tunnel: [w600 w632] -> w563
                tunnel: w562 -> [w599 _]
                tunnel: w561 -> [w598 w633]
                tunnel: [w579 UtilityLib.valueStatus."no info available" ("valueStatus")] -> w559
                tunnel: [w578 w629] -> w558
                tunnel: w555 -> [w576 w630]
                tunnel: w554 -> [w575 w631]
                tunnel: w552 -> [w574 _]
                tunnel: w553 -> [_ w629]
                tunnel: 1 -> [w572 _]
                tunnel: -1.0 -> [w571 _]
                frame False {
                  n178 = Type Cast(x=w599) -> (*(type *) &x=w577:string)  [unwired: 1 in]
                  n179 = case shown="True" w574 {
                    tunnel: [w615 w625] -> w589
                    tunnel: [w614 w624] -> w588
                    tunnel: [w613 w623] -> w587
                    tunnel: [w612 w618] -> w586
                    tunnel: [w611 w618] -> w585
                    tunnel: [w610 w618] -> w584
                    tunnel: [w609 w622] -> w597
                    tunnel: [w608 w621] -> w596
                    tunnel: [w607 w620] -> w595
                    tunnel: [w606 w617] -> w594
                    tunnel: [w605 w617] -> w593
                    tunnel: [w604 w617] -> w592
                    tunnel: w577 -> [w601 w619]
                    tunnel: w572 -> [w603 w617]
                    tunnel: w571 -> [w602 w618]
                    frame True {
                      n180 = Scan From String(format string="%d:%f:%d:%f:%d:%f:%d:%f:%d:%f:%d:%f", input string=w601, default 1=w603, default 2=w602, default 3=w603, default 4=w602, default 5=w603, default 6=w602, default 7=w603, default 8=w602, default 9=w603, default 10=w602, default 11=w603, default 12=w602) -> (output 1=w609:i32, output 2=w615:dbl, output 3=w608:i32, output 4=w614:dbl, output 5=w607:i32, output 6=w613:dbl, output 7=w606:i32, output 8=w612:dbl, output 9=w605:i32, output 10=w611:dbl, output 11=w604:i32, output 12=w610:dbl)  [unwired: 2 in, 3 out]
                    }
                    frame False {
                      n181 = Scan From String(format string="%d:%f:%d:%f:%d:%f", input string=w619, default 1=w617, default 2=w618, default 3=w617, default 4=w618, default 5=w617, default 6=w618) -> (output 1=w622:i32, output 2=w625:dbl, output 3=w621:i32, output 4=w624:dbl, output 5=w620:i32, output 6=w623:dbl)  [unwired: 2 in, 3 out]
                    }
                  }
                  n182 = Bundle By Name(cluster=w598, "FanStat.DIM Status.quality"=w575, "FanStat.DIM Status.Time Stamp"=w576, "FanStat.FanStat"=w577, "FanStat.DIM Status.no link"=w573) -> (w600:T7)
                  n183 = Build Array(w597, w596, w595, w594, w593, w592) -> (w591:i32[])
                  n184 = Greater Than 0?(x=w591) -> (x > 0?=w590:bool[])
                  n185 = Build Array(w589, w588, w587, w586, w585, w584) -> (w583:dbl[])
                  n186 = Or Array Elements(Boolean array=w590) -> (logical OR=w582:bool)
                  n187 = Type Cast(x=w583) -> (*(type *) &x=w578:string)  [unwired: 1 in]
                  n188 = Select(t=UtilityLib.valueStatus."on" ("valueStatus"), s=w582, f=UtilityLib.valueStatus."alarm/malfunction" ("valueStatus")) -> (s? t:f=w579:T4)
                }
                frame True {
                  n189 = Bundle By Name(cluster=w633, "FanStat.DIM Status.quality"=w631, "FanStat.DIM Status.Time Stamp"=w630, "FanStat.DIM Status.no link"=w628) -> (w632:T7)
                }
              }
              n190 = call "CAEN_HVSystem.set modified data.vi"("i ref in"=w567, "i attribute"=w563, "error in (no error)"=w566) -> ("i ref out"=w564:refnum<vi>, "error out"=w565:errorcluster)  [unwired: 15 in]
            }
            frame Error {
              n191 = call "CoreLib.set data type mismatch.vi"("error in (no error)"=w637, "error source"=w635) -> ("error out"=w636:errorcluster)  [unwired: 17 in]
            }
          }
          n192 = call "BaseProcess.set event status.vi"("i ref in"=w543, "EventStatus"=w540, "error in (no error)"=w542) -> ("i ref out"=w529:refnum<vi>, "error out"=w541:errorcluster)  [unwired: 14 in, 1 out]
          n193 = Unbundle By Name(w541) -> ("source"=w535:string, "code"=w547:i32)
          n194 = call "CAEN_HVSystem.get i attribute.vi"("i ref in"=w529) -> ("i ref out"=w528:refnum<vi>, "i attribute"=w533:T7)  [unwired: 16 in, 1 out]
          n195 = Unbundle By Name(w533) -> ("DIM Service IDs.Fan Status"=w527:i32)
          n196 = call "LVDimInterface.dis_set_quality.vi"("my_serviceID"=w527, "quality"=w521) -> ("my_serviceID (out)"=w530:i32, "error out"=w525:errorcluster)  [unwired: 16 in]
          n197 = call-poly "CoreLib.data 2 byte array.vi"("string"=w535) -> ("byteArray out"=w544:T1)  [unwired: 18 in]
          n198 = call "LVDimInterface.dis_update_service.vi"("my_serviceID"=w530, "data"=w520, "error in (no error)"=w525) -> ()  [unwired: 14 in, 3 out]
          n199 = Bundle By Name(cluster=w546, "Data"=w544, "Error #"=w547, "Data Descriptor"="C:N") -> (w545:T2)
        }
        frame "HVClkConf" {
          n200 = call "CAEObj.unfold trend data.vi"("i ref in"=w647, "raw trend data"=w648) -> ("quality"=w641:i32, "timeStamp"=w642:dbl, "no link"=w639:bool, "i ref out"=w646:refnum<vi>, "data"=w645:i8[], "typeDescriptor"=w643:string, "error out"=w640:errorcluster)  [unwired: 9 in, 2 out]
          n201 = case shown="No Error" w640 {
            tunnel: [w667 w690] -> w655
            tunnel: w646 -> [w674 w690]
            tunnel: w660 -> [w673 w689]
            tunnel: [w668 w688] -> w654
            tunnel: w652 -> [_ w687]
            tunnel: w649 -> [w672 _]
            tunnel: w645 -> [w665 _]
            tunnel: w643 -> [_ _]
            tunnel: w642 -> [w663 _]
            tunnel: w641 -> [w662 _]
            tunnel: w639 -> [w661 _]
            frame No Error {
              n202 = To Time Stamp(1:w663) -> (0:w664:timestamp)
              n203 = call "CAEN_HVSystem.get data to modify.vi"("i ref in"=w674, "ms timeout (10000)"=w672, "error in (no error)"=w673) -> ("i ref out"=w670:refnum<vi>, "i attribute"=w671:T7, "error out"=w669:errorcluster)  [unwired: 13 in, 1 out]
              n204 = case "no link?" shown="False" w661 {
                selector: w661 -> [w675 w680]
                tunnel: w671 -> [w679 w686]
                tunnel: [w678 w685] -> w666
                tunnel: w665 -> [_ w684]
                tunnel: w664 -> [w677 w682]
                tunnel: w662 -> [w676 w681]
                frame True {
                  n205 = Bundle By Name(cluster=w679, "HVClkConf.DIM Status.quality"=w676, "HVClkConf.DIM Status.Time Stamp"=w677, "HVClkConf.DIM Status.no link"=w675) -> (w678:T7)
                }
                frame False {
                  n206 = Type Cast(x=w684) -> (*(type *) &x=w683:string)  [unwired: 1 in]
                  n207 = Bundle By Name(cluster=w686, "HVClkConf.DIM Status.quality"=w681, "HVClkConf.DIM Status.Time Stamp"=w682, "HVClkConf.HVClkConf"=w683, "HVClkConf.DIM Status.no link"=w680) -> (w685:T7)
                }
              }
              n208 = call "CAEN_HVSystem.set modified data.vi"("i ref in"=w670, "i attribute"=w666, "error in (no error)"=w669) -> ("i ref out"=w667:refnum<vi>, "error out"=w668:errorcluster)  [unwired: 15 in]
            }
            frame Error {
              n209 = call "CoreLib.set data type mismatch.vi"("error in (no error)"=w689, "error source"=w687) -> ("error out"=w688:errorcluster)  [unwired: 17 in]
            }
          }
          n210 = call "BaseProcess.set event status.vi"("i ref in"=w655, "EventStatus"=w652, "error in (no error)"=w654) -> ("i ref out"=w651:refnum<vi>, "error out"=w653:errorcluster)  [unwired: 14 in, 1 out]
          n211 = Unbundle By Name(w653) -> ("source"=w644:string, "code"=w659:i32)
          n212 = call-poly "CoreLib.data 2 byte array.vi"("string"=w644) -> ("byteArray out"=w656:T1)  [unwired: 18 in]
          n213 = Bundle By Name(cluster=w658, "Data"=w656, "Error #"=w659, "Data Descriptor"="C:N") -> (w657:T2)
        }
        frame "IPAddr" {
          n214 = call "CAEObj.unfold trend data.vi"("i ref in"=w699, "raw trend data"=w700) -> ("quality"=w694:i32, "timeStamp"=w693:dbl, "no link"=w691:bool, "i ref out"=w698:refnum<vi>, "data"=w697:i8[], "typeDescriptor"=w695:string, "error out"=w692:errorcluster)  [unwired: 9 in, 2 out]
          n215 = case shown="No Error" w692 {
            tunnel: [w725 w761] -> w707
            tunnel: w698 -> [w732 w761]
            tunnel: w712 -> [w731 w760]
            tunnel: [w724 w759] -> w706
            tunnel: w704 -> [_ w758]
            tunnel: w701 -> [w730 _]
            tunnel: w697 -> [w726 _]
            tunnel: w695 -> [_ _]
            tunnel: w694 -> [w717 _]
            tunnel: w693 -> [w716 _]
            tunnel: w691 -> [w714 _]
            frame No Error {
              n216 = To Time Stamp(1:w716) -> (0:w715:timestamp)
              n217 = call "CAEN_HVSystem.get data to modify.vi"("i ref in"=w732, "ms timeout (10000)"=w730, "error in (no error)"=w731) -> ("i ref out"=w729:refnum<vi>, "i attribute"=w721:T7, "error out"=w728:errorcluster)  [unwired: 13 in, 1 out]
              n218 = Unbundle By Name(w721) -> ("System Name"=w720:string, "ModelName.ModelName"=w719:string)
              n219 = case "no link?" shown="False" w714 {
                selector: w714 -> [w746 w753]
                tunnel: [w752 w757] -> w727
                tunnel: w726 -> [w751 _]
                tunnel: w721 -> [w750 w756]
                tunnel: [w749 _] -> w718
                tunnel: w717 -> [w748 w755]
                tunnel: w715 -> [w747 w754]
                tunnel: [w746 w753] -> w713
                frame False {
                  n220 = Type Cast(x=w751) -> (*(type *) &x=w749:string)  [unwired: 1 in]
                  n221 = Bundle By Name(cluster=w750, "IPAddr.DIM Status.quality"=w748, "IPAddr.DIM Status.Time Stamp"=w747, "IPAddr.IPAddr"=w749, "IPAddr.DIM Status.no link"=w746) -> (w752:T7)
                }
                frame True {
                  n222 = Bundle By Name(cluster=w756, "IPAddr.DIM Status.quality"=w755, "IPAddr.DIM Status.Time Stamp"=w754, "IPAddr.DIM Status.no link"=w753) -> (w757:T7)
                }
              }
              n223 = call "CAEN_HVSystem.set modified data.vi"("i ref in"=w729, "i attribute"=w727, "error in (no error)"=w728) -> ("i ref out"=w722:refnum<vi>, "error out"=w723:errorcluster)  [unwired: 15 in]
              n224 = case "no link?" shown="False" w713 {
                tunnel: [w739 w745] -> w725
                tunnel: [w738 w744] -> w724
                tunnel: w723 -> [w737 w744]
                tunnel: w722 -> [w736 w745]
                tunnel: w720 -> [w735 _]
                tunnel: w719 -> [w734 _]
                tunnel: w718 -> [w733 _]
                frame False {
                  n225 = Concatenate Strings("CAEN HV System: " ("string"), w735, "; Model: " ("string"), w734, "IP: " ("string"), w733) -> (w743:string)
                  n226 = call "DeviceBase.set device ID.vi"("i ref in"=w736, "deviceID"=w743, "error in (no error)"=w737) -> ("i ref out"=w739:refnum<vi>, "error out"=w738:errorcluster)  [unwired: 14 in, 1 out]
                }
                frame True {
                }
              }
            }
            frame Error {
              n227 = call "CoreLib.set data type mismatch.vi"("error in (no error)"=w760, "error source"=w758) -> ("error out"=w759:errorcluster)  [unwired: 17 in]
            }
          }
          n228 = call "BaseProcess.set event status.vi"("i ref in"=w707, "EventStatus"=w704, "error in (no error)"=w706) -> ("i ref out"=w703:refnum<vi>, "error out"=w705:errorcluster)  [unwired: 14 in, 1 out]
          n229 = Unbundle By Name(w705) -> ("source"=w696:string, "code"=w711:i32)
          n230 = call-poly "CoreLib.data 2 byte array.vi"("string"=w696) -> ("byteArray out"=w708:T1)  [unwired: 18 in]
          n231 = Bundle By Name(cluster=w710, "Data"=w708, "Error #"=w711, "Data Descriptor"="C:N") -> (w709:T2)
        }
        frame "IPNetMsk" {
          n232 = call "CAEObj.unfold trend data.vi"("i ref in"=w770, "raw trend data"=w771) -> ("quality"=w765:i32, "timeStamp"=w764:dbl, "no link"=w762:bool, "i ref out"=w769:refnum<vi>, "data"=w768:i8[], "typeDescriptor"=w766:string, "error out"=w763:errorcluster)  [unwired: 9 in, 2 out]
          n233 = case shown="No Error" w763 {
            tunnel: [w790 w813] -> w778
            tunnel: w769 -> [w797 w813]
            tunnel: w783 -> [w796 w812]
            tunnel: [w791 w811] -> w777
            tunnel: w775 -> [_ w810]
            tunnel: w772 -> [w795 _]
            tunnel: w768 -> [w788 _]
            tunnel: w766 -> [_ _]
            tunnel: w765 -> [w787 _]
            tunnel: w764 -> [w785 _]
            tunnel: w762 -> [w784 _]
            frame No Error {
              n234 = call "CAEN_HVSystem.get data to modify.vi"("i ref in"=w797, "ms timeout (10000)"=w795, "error in (no error)"=w796) -> ("i ref out"=w793:refnum<vi>, "i attribute"=w794:T7, "error out"=w792:errorcluster)  [unwired: 13 in, 1 out]
              n235 = To Time Stamp(1:w785) -> (0:w786:timestamp)
              n236 = case "no link?" shown="False" w784 {
                selector: w784 -> [w798 w805]
                tunnel: w794 -> [w804 w809]
                tunnel: [w803 w808] -> w789
                tunnel: w788 -> [w802 _]
                tunnel: w787 -> [w800 w807]
                tunnel: w786 -> [w799 w806]
                frame False {
                  n237 = Type Cast(x=w802) -> (*(type *) &x=w801:string)  [unwired: 1 in]
                  n238 = Bundle By Name(cluster=w804, "IPNetMsk.DIM Status.quality"=w800, "IPNetMsk.DIM Status.Time Stamp"=w799, "IPNetMsk.IPNetMsk"=w801, "IPNetMsk.DIM Status.no link"=w798) -> (w803:T7)
                }
                frame True {
                  n239 = Bundle By Name(cluster=w809, "IPNetMsk.DIM Status.quality"=w807, "IPNetMsk.DIM Status.Time Stamp"=w806, "IPNetMsk.DIM Status.no link"=w805) -> (w808:T7)
                }
              }
              n240 = call "CAEN_HVSystem.set modified data.vi"("i ref in"=w793, "i attribute"=w789, "error in (no error)"=w792) -> ("i ref out"=w790:refnum<vi>, "error out"=w791:errorcluster)  [unwired: 15 in]
            }
            frame Error {
              n241 = call "CoreLib.set data type mismatch.vi"("error in (no error)"=w812, "error source"=w810) -> ("error out"=w811:errorcluster)  [unwired: 17 in]
            }
          }
          n242 = call "BaseProcess.set event status.vi"("i ref in"=w778, "EventStatus"=w775, "error in (no error)"=w777) -> ("i ref out"=w774:refnum<vi>, "error out"=w776:errorcluster)  [unwired: 14 in, 1 out]
          n243 = Unbundle By Name(w776) -> ("source"=w767:string, "code"=w782:i32)
          n244 = call-poly "CoreLib.data 2 byte array.vi"("string"=w767) -> ("byteArray out"=w779:T1)  [unwired: 18 in]
          n245 = Bundle By Name(cluster=w781, "Data"=w779, "Error #"=w782, "Data Descriptor"="C:N") -> (w780:T2)
        }
        frame "IPGw" {
          n246 = call "CAEObj.unfold trend data.vi"("i ref in"=w822, "raw trend data"=w823) -> ("quality"=w815:i32, "timeStamp"=w814:dbl, "no link"=w816:bool, "i ref out"=w821:refnum<vi>, "data"=w820:i8[], "typeDescriptor"=w818:string, "error out"=w817:errorcluster)  [unwired: 9 in, 2 out]
          n247 = case shown="No Error" w817 {
            tunnel: [w842 w865] -> w830
            tunnel: w821 -> [w849 w865]
            tunnel: w835 -> [w848 w864]
            tunnel: [w843 w863] -> w829
            tunnel: w827 -> [_ w862]
            tunnel: w824 -> [w847 _]
            tunnel: w820 -> [w840 _]
            tunnel: w818 -> [_ _]
            tunnel: w816 -> [w836 _]
            tunnel: w815 -> [w839 _]
            tunnel: w814 -> [w838 _]
            frame No Error {
              n248 = To Time Stamp(1:w838) -> (0:w837:timestamp)
              n249 = call "CAEN_HVSystem.get data to modify.vi"("i ref in"=w849, "ms timeout (10000)"=w847, "error in (no error)"=w848) -> ("i ref out"=w845:refnum<vi>, "i attribute"=w846:T7, "error out"=w844:errorcluster)  [unwired: 13 in, 1 out]
              n250 = case "no link?" shown="False" w836 {
                selector: w836 -> [w850 w857]
                tunnel: w846 -> [w856 w861]
                tunnel: [w855 w860] -> w841
                tunnel: w840 -> [w854 _]
                tunnel: w839 -> [w852 w859]
                tunnel: w837 -> [w851 w858]
                frame False {
                  n251 = Type Cast(x=w854) -> (*(type *) &x=w853:string)  [unwired: 1 in]
                  n252 = Bundle By Name(cluster=w856, "IPGw.DIM Status.quality"=w852, "IPGw.DIM Status.Time Stamp"=w851, "IPGw.IPGw"=w853, "IPGw.DIM Status.no link"=w850) -> (w855:T7)
                }
                frame True {
                  n253 = Bundle By Name(cluster=w861, "IPGw.DIM Status.quality"=w859, "IPGw.DIM Status.Time Stamp"=w858, "IPGw.DIM Status.no link"=w857) -> (w860:T7)
                }
              }
              n254 = call "CAEN_HVSystem.set modified data.vi"("i ref in"=w845, "i attribute"=w841, "error in (no error)"=w844) -> ("i ref out"=w842:refnum<vi>, "error out"=w843:errorcluster)  [unwired: 15 in]
            }
            frame Error {
              n255 = call "CoreLib.set data type mismatch.vi"("error in (no error)"=w864, "error source"=w862) -> ("error out"=w863:errorcluster)  [unwired: 17 in]
            }
          }
          n256 = call "BaseProcess.set event status.vi"("i ref in"=w830, "EventStatus"=w827, "error in (no error)"=w829) -> ("i ref out"=w826:refnum<vi>, "error out"=w828:errorcluster)  [unwired: 14 in, 1 out]
          n257 = Unbundle By Name(w828) -> ("source"=w819:string, "code"=w834:i32)
          n258 = call-poly "CoreLib.data 2 byte array.vi"("string"=w819) -> ("byteArray out"=w831:T1)  [unwired: 18 in]
          n259 = Bundle By Name(cluster=w833, "Data"=w831, "Error #"=w834, "Data Descriptor"="C:N") -> (w832:T2)
        }
        frame "RS232Par" {
          n260 = call "CAEObj.unfold trend data.vi"("i ref in"=w874, "raw trend data"=w875) -> ("quality"=w869:i32, "timeStamp"=w868:dbl, "no link"=w866:bool, "i ref out"=w873:refnum<vi>, "data"=w872:i8[], "typeDescriptor"=w870:string, "error out"=w867:errorcluster)  [unwired: 9 in, 2 out]
          n261 = case shown="No Error" w867 {
            tunnel: [w894 w917] -> w882
            tunnel: w873 -> [w901 w917]
            tunnel: w887 -> [w900 w916]
            tunnel: [w895 w915] -> w881
            tunnel: w879 -> [_ w914]
            tunnel: w876 -> [w899 _]
            tunnel: w872 -> [w892 _]
            tunnel: w870 -> [_ _]
            tunnel: w869 -> [w891 _]
            tunnel: w868 -> [w890 _]
            tunnel: w866 -> [w888 _]
            frame No Error {
              n262 = To Time Stamp(1:w890) -> (0:w889:timestamp)
              n263 = call "CAEN_HVSystem.get data to modify.vi"("i ref in"=w901, "ms timeout (10000)"=w899, "error in (no error)"=w900) -> ("i ref out"=w897:refnum<vi>, "i attribute"=w898:T7, "error out"=w896:errorcluster)  [unwired: 13 in, 1 out]
              n264 = case "no link?" shown="False" w888 {
                selector: w888 -> [w902 w907]
                tunnel: w898 -> [w906 w913]
                tunnel: [w905 w912] -> w893
                tunnel: w892 -> [_ w911]
                tunnel: w891 -> [w904 w909]
                tunnel: w889 -> [w903 w908]
                frame True {
                  n265 = Bundle By Name(cluster=w906, "RS232Par.DIM Status.quality"=w904, "RS232Par.DIM Status.Time Stamp"=w903, "RS232Par.DIM Status.no link"=w902) -> (w905:T7)
                }
                frame False {
                  n266 = Type Cast(x=w911) -> (*(type *) &x=w910:string)  [unwired: 1 in]
                  n267 = Bundle By Name(cluster=w913, "RS232Par.DIM Status.quality"=w909, "RS232Par.DIM Status.Time Stamp"=w908, "RS232Par.RS232Par"=w910, "RS232Par.DIM Status.no link"=w907) -> (w912:T7)
                }
              }
              n268 = call "CAEN_HVSystem.set modified data.vi"("i ref in"=w897, "i attribute"=w893, "error in (no error)"=w896) -> ("i ref out"=w894:refnum<vi>, "error out"=w895:errorcluster)  [unwired: 15 in]
            }
            frame Error {
              n269 = call "CoreLib.set data type mismatch.vi"("error in (no error)"=w916, "error source"=w914) -> ("error out"=w915:errorcluster)  [unwired: 17 in]
            }
          }
          n270 = call "BaseProcess.set event status.vi"("i ref in"=w882, "EventStatus"=w879, "error in (no error)"=w881) -> ("i ref out"=w878:refnum<vi>, "error out"=w880:errorcluster)  [unwired: 14 in, 1 out]
          n271 = Unbundle By Name(w880) -> ("source"=w871:string, "code"=w886:i32)
          n272 = call-poly "CoreLib.data 2 byte array.vi"("string"=w871) -> ("byteArray out"=w883:T1)  [unwired: 18 in]
          n273 = Bundle By Name(cluster=w885, "Data"=w883, "Error #"=w886, "Data Descriptor"="C:N") -> (w884:T2)
        }
        frame "Slots" {
          n274 = call "CAEObj.unfold trend data.vi"("i ref in"=w926, "raw trend data"=w927) -> ("quality"=w921:i32, "timeStamp"=w920:dbl, "no link"=w918:bool, "i ref out"=w925:refnum<vi>, "data"=w924:i8[], "typeDescriptor"=w922:string, "error out"=w919:errorcluster)  [unwired: 9 in, 2 out]
          n275 = case shown="No Error" w919 {
            tunnel: [w946 w971] -> w934
            tunnel: w925 -> [w953 w971]
            tunnel: w939 -> [w952 w970]
            tunnel: [w947 w969] -> w933
            tunnel: w931 -> [_ w968]
            tunnel: w928 -> [w951 _]
            tunnel: w924 -> [w944 _]
            tunnel: w922 -> [_ _]
            tunnel: w921 -> [w943 _]
            tunnel: w920 -> [w942 _]
            tunnel: w918 -> [w940 _]
            frame No Error {
              n276 = call "CAEN_HVSystem.get data to modify.vi"("i ref in"=w953, "ms timeout (10000)"=w951, "error in (no error)"=w952) -> ("i ref out"=w949:refnum<vi>, "i attribute"=w950:T7, "error out"=w948:errorcluster)  [unwired: 13 in, 1 out]
              n277 = To Time Stamp(1:w942) -> (0:w941:timestamp)
              n278 = case "no link?" shown="False" w940 {
                selector: w940 -> [w954 w959]
                tunnel: w950 -> [w958 w967]
                tunnel: [w957 w966] -> w945
                tunnel: w944 -> [_ w964]
                tunnel: w943 -> [w956 w961]
                tunnel: w941 -> [w955 w960]
                frame True {
                  n279 = Bundle By Name(cluster=w958, "Slots.DIM Status.quality"=w956, "Slots.DIM Status.Time Stamp"=w955, "Slots.DIM Status.no link"=w954) -> (w957:T7)
                }
                frame False {
                  w963 = 0.0  # Dbl
                  n280 = Type Cast(type=w963, x=w964) -> (*(type *) &x=w965:dbl)
                  n281 = To Word Integer(number=w965) -> (16bit integer=w962:i16)
                  n282 = Bundle By Name(cluster=w967, "Slots.DIM Status.quality"=w961, "Slots.DIM Status.Time Stamp"=w960, "Slots.Slots"=w962, "Slots.DIM Status.no link"=w959) -> (w966:T7)
                }
              }
              n283 = call "CAEN_HVSystem.set modified data.vi"("i ref in"=w949, "i attribute"=w945, "error in (no error)"=w948) -> ("i ref out"=w946:refnum<vi>, "error out"=w947:errorcluster)  [unwired: 15 in]
            }
            frame Error {
              n284 = call "CoreLib.set data type mismatch.vi"("error in (no error)"=w970, "error source"=w968) -> ("error out"=w969:errorcluster)  [unwired: 17 in]
            }
          }
          n285 = call "BaseProcess.set event status.vi"("i ref in"=w934, "EventStatus"=w931, "error in (no error)"=w933) -> ("i ref out"=w930:refnum<vi>, "error out"=w932:errorcluster)  [unwired: 14 in, 1 out]
          n286 = Unbundle By Name(w932) -> ("source"=w923:string, "code"=w938:i32)
          n287 = call-poly "CoreLib.data 2 byte array.vi"("string"=w923) -> ("byteArray out"=w935:T1)  [unwired: 18 in]
          n288 = Bundle By Name(cluster=w937, "Data"=w935, "Error #"=w938, "Data Descriptor"="C:N") -> (w936:T2)
        }
        frame "GenSignCfg" {
          n289 = call "CAEObj.unfold trend data.vi"("i ref in"=w980, "raw trend data"=w981) -> ("quality"=w975:i32, "timeStamp"=w974:dbl, "no link"=w972:bool, "i ref out"=w979:refnum<vi>, "data"=w978:i8[], "typeDescriptor"=w976:string, "error out"=w973:errorcluster)  [unwired: 9 in, 2 out]
          n290 = case shown="No Error" w973 {
            tunnel: [w1000 w1025] -> w988
            tunnel: w979 -> [w1007 w1025]
            tunnel: w993 -> [w1006 w1024]
            tunnel: [w1001 w1023] -> w987
            tunnel: w985 -> [_ w1022]
            tunnel: w982 -> [w1005 _]
            tunnel: w978 -> [w998 _]
            tunnel: w976 -> [_ _]
            tunnel: w975 -> [w997 _]
            tunnel: w974 -> [w996 _]
            tunnel: w972 -> [w994 _]
            frame No Error {
              n291 = To Time Stamp(1:w996) -> (0:w995:timestamp)
              n292 = call "CAEN_HVSystem.get data to modify.vi"("i ref in"=w1007, "ms timeout (10000)"=w1005, "error in (no error)"=w1006) -> ("i ref out"=w1003:refnum<vi>, "i attribute"=w1004:T7, "error out"=w1002:errorcluster)  [unwired: 13 in, 1 out]
              n293 = case "no link?" shown="False" w994 {
                selector: w994 -> [w1008 w1013]
                tunnel: w1004 -> [w1012 w1021]
                tunnel: [w1011 w1020] -> w999
                tunnel: w998 -> [_ w1018]
                tunnel: w997 -> [w1010 w1015]
                tunnel: w995 -> [w1009 w1014]
                frame True {
                  n294 = Bundle By Name(cluster=w1012, "GenSignCfg.DIM Status.quality"=w1010, "GenSignCfg.DIM Status.Time Stamp"=w1009, "GenSignCfg.DIM Status.no link"=w1008) -> (w1011:T7)
                }
                frame False {
                  w1017 = 0.0  # Dbl
                  n295 = Type Cast(type=w1017, x=w1018) -> (*(type *) &x=w1019:dbl)
                  n296 = To Word Integer(number=w1019) -> (16bit integer=w1016:i16)
                  n297 = Bundle By Name(cluster=w1021, "GenSignCfg.DIM Status.quality"=w1015, "GenSignCfg.DIM Status.Time Stamp"=w1014, "GenSignCfg.GenSignCfg"=w1016, "GenSignCfg.DIM Status.no link"=w1013) -> (w1020:T7)
                }
              }
              n298 = call "CAEN_HVSystem.set modified data.vi"("i ref in"=w1003, "i attribute"=w999, "error in (no error)"=w1002) -> ("i ref out"=w1000:refnum<vi>, "error out"=w1001:errorcluster)  [unwired: 15 in]
            }
            frame Error {
              n299 = call "CoreLib.set data type mismatch.vi"("error in (no error)"=w1024, "error source"=w1022) -> ("error out"=w1023:errorcluster)  [unwired: 17 in]
            }
          }
          n300 = call "BaseProcess.set event status.vi"("i ref in"=w988, "EventStatus"=w985, "error in (no error)"=w987) -> ("i ref out"=w984:refnum<vi>, "error out"=w986:errorcluster)  [unwired: 14 in, 1 out]
          n301 = Unbundle By Name(w986) -> ("source"=w977:string, "code"=w992:i32)
          n302 = call-poly "CoreLib.data 2 byte array.vi"("string"=w977) -> ("byteArray out"=w989:T1)  [unwired: 18 in]
          n303 = Bundle By Name(cluster=w991, "Data"=w989, "Error #"=w992, "Data Descriptor"="C:N") -> (w990:T2)
        }
        frame "FrontPanIn" {
          n304 = call "CAEObj.unfold trend data.vi"("i ref in"=w1034, "raw trend data"=w1035) -> ("quality"=w1029:i32, "timeStamp"=w1028:dbl, "no link"=w1026:bool, "i ref out"=w1033:refnum<vi>, "data"=w1032:i8[], "typeDescriptor"=w1030:string, "error out"=w1027:errorcluster)  [unwired: 9 in, 2 out]
          n305 = case shown="No Error" w1027 {
            tunnel: [w1054 w1079] -> w1042
            tunnel: w1033 -> [w1061 w1079]
            tunnel: w1047 -> [w1060 w1078]
            tunnel: [w1055 w1077] -> w1041
            tunnel: w1039 -> [_ w1076]
            tunnel: w1036 -> [w1059 _]
            tunnel: w1032 -> [w1052 _]
            tunnel: w1030 -> [_ _]
            tunnel: w1029 -> [w1051 _]
            tunnel: w1028 -> [w1049 _]
            tunnel: w1026 -> [w1048 _]
            frame No Error {
              n306 = To Time Stamp(1:w1049) -> (0:w1050:timestamp)
              n307 = call "CAEN_HVSystem.get data to modify.vi"("i ref in"=w1061, "ms timeout (10000)"=w1059, "error in (no error)"=w1060) -> ("i ref out"=w1057:refnum<vi>, "i attribute"=w1058:T7, "error out"=w1056:errorcluster)  [unwired: 13 in, 1 out]
              n308 = case "no link?" shown="False" w1048 {
                selector: w1048 -> [w1062 w1067]
                tunnel: w1058 -> [w1066 w1075]
                tunnel: [w1065 w1074] -> w1053
                tunnel: w1052 -> [_ w1072]
                tunnel: w1051 -> [w1064 w1069]
                tunnel: w1050 -> [w1063 w1068]
                frame True {
                  n309 = Bundle By Name(cluster=w1066, "FrontPanIn.DIM Status.quality"=w1064, "FrontPanIn.DIM Status.Time Stamp"=w1063, "FrontPanIn.DIM Status.no link"=w1062) -> (w1065:T7)
                }
                frame False {
                  w1071 = 0.0  # Dbl
                  n310 = Type Cast(type=w1071, x=w1072) -> (*(type *) &x=w1073:dbl)
                  n311 = To Word Integer(number=w1073) -> (16bit integer=w1070:i16)
                  n312 = Bundle By Name(cluster=w1075, "FrontPanIn.DIM Status.quality"=w1069, "FrontPanIn.DIM Status.Time Stamp"=w1068, "FrontPanIn.FrontPanIn"=w1070, "FrontPanIn.DIM Status.no link"=w1067) -> (w1074:T7)
                }
              }
              n313 = call "CAEN_HVSystem.set modified data.vi"("i ref in"=w1057, "i attribute"=w1053, "error in (no error)"=w1056) -> ("i ref out"=w1054:refnum<vi>, "error out"=w1055:errorcluster)  [unwired: 15 in]
            }
            frame Error {
              n314 = call "CoreLib.set data type mismatch.vi"("error in (no error)"=w1078, "error source"=w1076) -> ("error out"=w1077:errorcluster)  [unwired: 17 in]
            }
          }
          n315 = call "BaseProcess.set event status.vi"("i ref in"=w1042, "EventStatus"=w1039, "error in (no error)"=w1041) -> ("i ref out"=w1038:refnum<vi>, "error out"=w1040:errorcluster)  [unwired: 14 in, 1 out]
          n316 = Unbundle By Name(w1040) -> ("source"=w1031:string, "code"=w1046:i32)
          n317 = call-poly "CoreLib.data 2 byte array.vi"("string"=w1031) -> ("byteArray out"=w1043:T1)  [unwired: 18 in]
          n318 = Bundle By Name(cluster=w1045, "Data"=w1043, "Error #"=w1046, "Data Descriptor"="C:N") -> (w1044:T2)
        }
        frame "FrontPanOut" {
          n319 = call "CAEObj.unfold trend data.vi"("i ref in"=w1088, "raw trend data"=w1089) -> ("quality"=w1083:i32, "timeStamp"=w1082:dbl, "no link"=w1080:bool, "i ref out"=w1087:refnum<vi>, "data"=w1086:i8[], "typeDescriptor"=w1084:string, "error out"=w1081:errorcluster)  [unwired: 9 in, 2 out]
          n320 = case shown="No Error" w1081 {
            tunnel: [w1108 w1145] -> w1096
            tunnel: w1087 -> [w1120 w1145]
            tunnel: w1101 -> [w1119 w1144]
            tunnel: [w1116 w1143] -> w1095
            tunnel: w1093 -> [_ w1142]
            tunnel: w1090 -> [w1118 _]
            tunnel: w1086 -> [w1114 _]
            tunnel: w1084 -> [_ _]
            tunnel: w1083 -> [w1113 _]
            tunnel: w1082 -> [w1112 _]
            tunnel: w1080 -> [w1110 _]
            frame No Error {
              n321 = To Time Stamp(1:w1112) -> (0:w1111:timestamp)
              n322 = call "CAEN_HVSystem.get data to modify.vi"("i ref in"=w1120, "ms timeout (10000)"=w1118, "error in (no error)"=w1119) -> ("i ref out"=w1106:refnum<vi>, "i attribute"=w1117:T7, "error out"=w1105:errorcluster)  [unwired: 13 in, 1 out]
              n323 = call "DeviceBase.get i attribute.vi"("i ref in"=w1106, "error in (no error)"=w1105) -> ("i attribute"=w1104:T8)  [unwired: 15 in, 2 out]
              n324 = Unbundle By Name(w1104) -> ("deviceState"=w1103:i32)
              n325 = case "no link?" shown="False" w1110 {
                selector: w1110 -> [w1122 w1134]
                tunnel: w1117 -> [w1126 w1141]
                tunnel: [w1125 w1140] -> w1115
                tunnel: w1114 -> [_ w1138]
                tunnel: w1113 -> [w1124 w1136]
                tunnel: w1111 -> [w1123 w1135]
                tunnel: [w1121 w1129] -> w1107
                tunnel: w1103 -> [w1121 w1127]
                frame True {
                  n326 = Bundle By Name(cluster=w1126, "FrontPanOut.DIM Status.quality"=w1124, "FrontPanOut.DIM Status.Time Stamp"=w1123, "FrontPanOut.DIM Status.no link"=w1122) -> (w1125:T7)
                }
                frame False {
                  w1130 = T9 -1 items=["ERROR"=-1, "OK"=0, "NOT_OK"=1] ("deviceState")
                  w1137 = 0.0  # Dbl
                  n327 = Type Cast(type=w1137, x=w1138) -> (*(type *) &x=w1139:dbl)
                  n328 = To Word Integer(number=w1139) -> (16bit integer=w1133:i16)
                  n329 = And(x=w1133, y=i16 775) -> (x .and. y?=w1131:i16)
                  n330 = Bundle By Name(cluster=w1141, "FrontPanOut.DIM Status.quality"=w1136, "FrontPanOut.DIM Status.Time Stamp"=w1135, "FrontPanOut.FrontPanOut"=w1133, "FrontPanOut.DIM Status.no link"=w1134) -> (w1140:T7)
                  n331 = Not Equal To 0?(x=w1131) -> (x != 0?=w1128:bool)
                  n332 = Select(t=w1130, s=w1128, f=w1127) -> (s? t:f=w1129:i32)
                }
              }
              n333 = call "CAEN_HVSystem.set modified data.vi"("i ref in"=w1106, "i attribute"=w1115, "error in (no error)"=w1105) -> ("i ref out"=w1109:refnum<vi>, "error out"=w1116:errorcluster)  [unwired: 15 in]
              n334 = call "DeviceBase.set device state.vi"("i ref in"=w1109, "deviceState"=w1107, "implicit"=FALSE) -> ("i ref out"=w1108:refnum<vi>)  [unwired: 14 in, 2 out]
            }
            frame Error {
              n335 = call "CoreLib.set data type mismatch.vi"("error in (no error)"=w1144, "error source"=w1142) -> ("error out"=w1143:errorcluster)  [unwired: 17 in]
            }
          }
          n336 = call "BaseProcess.set event status.vi"("i ref in"=w1096, "EventStatus"=w1093, "error in (no error)"=w1095) -> ("i ref out"=w1092:refnum<vi>, "error out"=w1094:errorcluster)  [unwired: 14 in, 1 out]
          n337 = Unbundle By Name(w1094) -> ("source"=w1085:string, "code"=w1100:i32)
          n338 = call-poly "CoreLib.data 2 byte array.vi"("string"=w1085) -> ("byteArray out"=w1097:T1)  [unwired: 18 in]
          n339 = Bundle By Name(cluster=w1099, "Data"=w1097, "Error #"=w1100, "Data Descriptor"="C:N") -> (w1098:T2)
        }
        frame "ClkFreq" {
          n340 = call "CAEObj.unfold trend data.vi"("i ref in"=w1154, "raw trend data"=w1155) -> ("quality"=w1149:i32, "timeStamp"=w1148:dbl, "no link"=w1146:bool, "i ref out"=w1153:refnum<vi>, "data"=w1152:i8[], "typeDescriptor"=w1150:string, "error out"=w1147:errorcluster)  [unwired: 9 in, 2 out]
          n341 = case shown="No Error" w1147 {
            tunnel: [w1174 w1199] -> w1162
            tunnel: w1153 -> [w1181 w1199]
            tunnel: w1167 -> [w1180 w1198]
            tunnel: [w1175 w1197] -> w1161
            tunnel: w1159 -> [_ w1196]
            tunnel: w1156 -> [w1179 _]
            tunnel: w1152 -> [w1172 _]
            tunnel: w1150 -> [_ _]
            tunnel: w1149 -> [w1171 _]
            tunnel: w1148 -> [w1170 _]
            tunnel: w1146 -> [w1168 _]
            frame No Error {
              n342 = To Time Stamp(1:w1170) -> (0:w1169:timestamp)
              n343 = call "CAEN_HVSystem.get data to modify.vi"("i ref in"=w1181, "ms timeout (10000)"=w1179, "error in (no error)"=w1180) -> ("i ref out"=w1177:refnum<vi>, "i attribute"=w1178:T7, "error out"=w1176:errorcluster)  [unwired: 13 in, 1 out]
              n344 = case "no link?" shown="False" w1168 {
                selector: w1168 -> [w1182 w1187]
                tunnel: w1178 -> [w1186 w1195]
                tunnel: [w1185 w1194] -> w1173
                tunnel: w1172 -> [_ w1192]
                tunnel: w1171 -> [w1184 w1189]
                tunnel: w1169 -> [w1183 w1188]
                frame True {
                  n345 = Bundle By Name(cluster=w1186, "ClkFreq.DIM Status.quality"=w1184, "ClkFreq.DIM Status.Time Stamp"=w1183, "ClkFreq.DIM Status.no link"=w1182) -> (w1185:T7)
                }
                frame False {
                  w1191 = 0.0  # Dbl
                  n346 = Type Cast(type=w1191, x=w1192) -> (*(type *) &x=w1193:dbl)
                  n347 = To Word Integer(number=w1193) -> (16bit integer=w1190:i16)
                  n348 = Bundle By Name(cluster=w1195, "ClkFreq.DIM Status.quality"=w1189, "ClkFreq.DIM Status.Time Stamp"=w1188, "ClkFreq.ClkFreq"=w1190, "ClkFreq.DIM Status.no link"=w1187) -> (w1194:T7)
                }
              }
              n349 = call "CAEN_HVSystem.set modified data.vi"("i ref in"=w1177, "i attribute"=w1173, "error in (no error)"=w1176) -> ("i ref out"=w1174:refnum<vi>, "error out"=w1175:errorcluster)  [unwired: 15 in]
            }
            frame Error {
              n350 = call "CoreLib.set data type mismatch.vi"("error in (no error)"=w1198, "error source"=w1196) -> ("error out"=w1197:errorcluster)  [unwired: 17 in]
            }
          }
          n351 = call "BaseProcess.set event status.vi"("i ref in"=w1162, "EventStatus"=w1159, "error in (no error)"=w1161) -> ("i ref out"=w1158:refnum<vi>, "error out"=w1160:errorcluster)  [unwired: 14 in, 1 out]
          n352 = Unbundle By Name(w1160) -> ("source"=w1151:string, "code"=w1166:i32)
          n353 = call-poly "CoreLib.data 2 byte array.vi"("string"=w1151) -> ("byteArray out"=w1163:T1)  [unwired: 18 in]
          n354 = Bundle By Name(cluster=w1165, "Data"=w1163, "Error #"=w1166, "Data Descriptor"="C:N") -> (w1164:T2)
        }
        frame "CnetCrNum" {
          n355 = call "CAEObj.unfold trend data.vi"("i ref in"=w1208, "raw trend data"=w1209) -> ("quality"=w1203:i32, "timeStamp"=w1202:dbl, "no link"=w1200:bool, "i ref out"=w1207:refnum<vi>, "data"=w1206:i8[], "typeDescriptor"=w1204:string, "error out"=w1201:errorcluster)  [unwired: 9 in, 2 out]
          n356 = case shown="No Error" w1201 {
            tunnel: [w1228 w1253] -> w1216
            tunnel: w1207 -> [w1235 w1253]
            tunnel: w1221 -> [w1234 w1252]
            tunnel: [w1229 w1251] -> w1215
            tunnel: w1213 -> [_ w1250]
            tunnel: w1210 -> [w1233 _]
            tunnel: w1206 -> [w1226 _]
            tunnel: w1204 -> [_ _]
            tunnel: w1203 -> [w1225 _]
            tunnel: w1202 -> [w1223 _]
            tunnel: w1200 -> [w1222 _]
            frame No Error {
              n357 = To Time Stamp(1:w1223) -> (0:w1224:timestamp)
              n358 = call "CAEN_HVSystem.get data to modify.vi"("i ref in"=w1235, "ms timeout (10000)"=w1233, "error in (no error)"=w1234) -> ("i ref out"=w1231:refnum<vi>, "i attribute"=w1232:T7, "error out"=w1230:errorcluster)  [unwired: 13 in, 1 out]
              n359 = case "no link?" shown="False" w1222 {
                selector: w1222 -> [w1236 w1241]
                tunnel: w1232 -> [w1240 w1249]
                tunnel: [w1239 w1248] -> w1227
                tunnel: w1226 -> [_ w1246]
                tunnel: w1225 -> [w1238 w1243]
                tunnel: w1224 -> [w1237 w1242]
                frame True {
                  n360 = Bundle By Name(cluster=w1240, "CnetCrNum.DIM Status.quality"=w1238, "CnetCrNum.DIM Status.Time Stamp"=w1237, "CnetCrNum.DIM Status.no link"=w1236) -> (w1239:T7)
                }
                frame False {
                  w1245 = 0.0  # Dbl
                  n361 = Type Cast(type=w1245, x=w1246) -> (*(type *) &x=w1247:dbl)
                  n362 = To Word Integer(number=w1247) -> (16bit integer=w1244:i16)
                  n363 = Bundle By Name(cluster=w1249, "CnetCrNum.DIM Status.quality"=w1243, "CnetCrNum.DIM Status.Time Stamp"=w1242, "CnetCrNum.CnetCrNum"=w1244, "CnetCrNum.DIM Status.no link"=w1241) -> (w1248:T7)
                }
              }
              n364 = call "CAEN_HVSystem.set modified data.vi"("i ref in"=w1231, "i attribute"=w1227, "error in (no error)"=w1230) -> ("i ref out"=w1228:refnum<vi>, "error out"=w1229:errorcluster)  [unwired: 15 in]
            }
            frame Error {
              n365 = call "CoreLib.set data type mismatch.vi"("error in (no error)"=w1252, "error source"=w1250) -> ("error out"=w1251:errorcluster)  [unwired: 17 in]
            }
          }
          n366 = call "BaseProcess.set event status.vi"("i ref in"=w1216, "EventStatus"=w1213, "error in (no error)"=w1215) -> ("i ref out"=w1212:refnum<vi>, "error out"=w1214:errorcluster)  [unwired: 14 in, 1 out]
          n367 = Unbundle By Name(w1214) -> ("source"=w1205:string, "code"=w1220:i32)
          n368 = call-poly "CoreLib.data 2 byte array.vi"("string"=w1205) -> ("byteArray out"=w1217:T1)  [unwired: 18 in]
          n369 = Bundle By Name(cluster=w1219, "Data"=w1217, "Error #"=w1220, "Data Descriptor"="C:N") -> (w1218:T2)
        }
        frame "Kill" {
          n370 = call "CAEObj.unfold trend data.vi"("i ref in"=w1262, "raw trend data"=w1263) -> ("quality"=w1257:i32, "timeStamp"=w1256:dbl, "no link"=w1254:bool, "i ref out"=w1261:refnum<vi>, "data"=w1260:i8[], "typeDescriptor"=w1258:string, "error out"=w1255:errorcluster)  [unwired: 9 in, 2 out]
          n371 = case shown="No Error" w1255 {
            tunnel: [w1282 w1307] -> w1270
            tunnel: w1261 -> [w1289 w1307]
            tunnel: w1275 -> [w1288 w1306]
            tunnel: [w1283 w1305] -> w1269
            tunnel: w1267 -> [_ w1304]
            tunnel: w1264 -> [w1287 _]
            tunnel: w1260 -> [w1280 _]
            tunnel: w1258 -> [_ _]
            tunnel: w1257 -> [w1279 _]
            tunnel: w1256 -> [w1277 _]
            tunnel: w1254 -> [w1276 _]
            frame No Error {
              n372 = To Time Stamp(1:w1277) -> (0:w1278:timestamp)
              n373 = call "CAEN_HVSystem.get data to modify.vi"("i ref in"=w1289, "ms timeout (10000)"=w1287, "error in (no error)"=w1288) -> ("i ref out"=w1285:refnum<vi>, "i attribute"=w1286:T7, "error out"=w1284:errorcluster)  [unwired: 13 in, 1 out]
              n374 = case "no link?" shown="False" w1276 {
                selector: w1276 -> [w1290 w1295]
                tunnel: w1286 -> [w1294 w1303]
                tunnel: [w1293 w1302] -> w1281
                tunnel: w1280 -> [_ w1300]
                tunnel: w1279 -> [w1292 w1297]
                tunnel: w1278 -> [w1291 w1296]
                frame True {
                  n375 = Bundle By Name(cluster=w1294, "Kill.DIM Status.quality"=w1292, "Kill.DIM Status.Time Stamp"=w1291, "Kill.DIM Status.no link"=w1290) -> (w1293:T7)
                }
                frame False {
                  w1299 = 0.0  # Dbl
                  n376 = Type Cast(type=w1299, x=w1300) -> (*(type *) &x=w1301:dbl)
                  n377 = Not Equal To 0?(x=w1301) -> (x != 0?=w1298:bool)
                  n378 = Bundle By Name(cluster=w1303, "Kill.DIM Status.quality"=w1297, "Kill.DIM Status.Time Stamp"=w1296, "Kill.Kill"=w1298, "Kill.DIM Status.no link"=w1295) -> (w1302:T7)
                }
              }
              n379 = call "CAEN_HVSystem.set modified data.vi"("i ref in"=w1285, "i attribute"=w1281, "error in (no error)"=w1284) -> ("i ref out"=w1282:refnum<vi>, "error out"=w1283:errorcluster)  [unwired: 15 in]
            }
            frame Error {
              n380 = call "CoreLib.set data type mismatch.vi"("error in (no error)"=w1306, "error source"=w1304) -> ("error out"=w1305:errorcluster)  [unwired: 17 in]
            }
          }
          n381 = call "BaseProcess.set event status.vi"("i ref in"=w1270, "EventStatus"=w1267, "error in (no error)"=w1269) -> ("i ref out"=w1266:refnum<vi>, "error out"=w1268:errorcluster)  [unwired: 14 in, 1 out]
          n382 = Unbundle By Name(w1268) -> ("source"=w1259:string, "code"=w1274:i32)
          n383 = call-poly "CoreLib.data 2 byte array.vi"("string"=w1259) -> ("byteArray out"=w1271:T1)  [unwired: 18 in]
          n384 = Bundle By Name(cluster=w1273, "Data"=w1271, "Error #"=w1274, "Data Descriptor"="C:N") -> (w1272:T2)
        }
        frame "ClearAlarm" {
          n385 = call "CAEObj.unfold trend data.vi"("i ref in"=w1316, "raw trend data"=w1317) -> ("quality"=w1311:i32, "timeStamp"=w1310:dbl, "no link"=w1308:bool, "i ref out"=w1315:refnum<vi>, "data"=w1314:i8[], "typeDescriptor"=w1312:string, "error out"=w1309:errorcluster)  [unwired: 9 in, 2 out]
          n386 = case shown="No Error" w1309 {
            tunnel: [w1336 w1361] -> w1324
            tunnel: w1315 -> [w1343 w1361]
            tunnel: w1329 -> [w1342 w1360]
            tunnel: [w1337 w1359] -> w1323
            tunnel: w1321 -> [_ w1358]
            tunnel: w1318 -> [w1341 _]
            tunnel: w1314 -> [w1334 _]
            tunnel: w1312 -> [_ _]
            tunnel: w1311 -> [w1333 _]
            tunnel: w1310 -> [w1331 _]
            tunnel: w1308 -> [w1330 _]
            frame No Error {
              n387 = To Time Stamp(1:w1331) -> (0:w1332:timestamp)
              n388 = call "CAEN_HVSystem.get data to modify.vi"("i ref in"=w1343, "ms timeout (10000)"=w1341, "error in (no error)"=w1342) -> ("i ref out"=w1339:refnum<vi>, "i attribute"=w1340:T7, "error out"=w1338:errorcluster)  [unwired: 13 in, 1 out]
              n389 = case "no link?" shown="False" w1330 {
                selector: w1330 -> [w1344 w1349]
                tunnel: w1340 -> [w1348 w1357]
                tunnel: [w1347 w1356] -> w1335
                tunnel: w1334 -> [_ w1354]
                tunnel: w1333 -> [w1346 w1351]
                tunnel: w1332 -> [w1345 w1350]
                frame True {
                  n390 = Bundle By Name(cluster=w1348, "ClearAlarm.DIM Status.quality"=w1346, "ClearAlarm.DIM Status.Time Stamp"=w1345, "ClearAlarm.DIM Status.no link"=w1344) -> (w1347:T7)
                }
                frame False {
                  w1353 = 0.0  # Dbl
                  n391 = Type Cast(type=w1353, x=w1354) -> (*(type *) &x=w1355:dbl)
                  n392 = Not Equal To 0?(x=w1355) -> (x != 0?=w1352:bool)
                  n393 = Bundle By Name(cluster=w1357, "ClearAlarm.DIM Status.quality"=w1351, "ClearAlarm.DIM Status.Time Stamp"=w1350, "ClearAlarm.ClearAlarm"=w1352, "ClearAlarm.DIM Status.no link"=w1349) -> (w1356:T7)
                }
              }
              n394 = call "CAEN_HVSystem.set modified data.vi"("i ref in"=w1339, "i attribute"=w1335, "error in (no error)"=w1338) -> ("i ref out"=w1336:refnum<vi>, "error out"=w1337:errorcluster)  [unwired: 15 in]
            }
            frame Error {
              n395 = call "CoreLib.set data type mismatch.vi"("error in (no error)"=w1360, "error source"=w1358) -> ("error out"=w1359:errorcluster)  [unwired: 17 in]
            }
          }
          n396 = call "BaseProcess.set event status.vi"("i ref in"=w1324, "EventStatus"=w1321, "error in (no error)"=w1323) -> ("i ref out"=w1320:refnum<vi>, "error out"=w1322:errorcluster)  [unwired: 14 in, 1 out]
          n397 = Unbundle By Name(w1322) -> ("source"=w1313:string, "code"=w1328:i32)
          n398 = call-poly "CoreLib.data 2 byte array.vi"("string"=w1313) -> ("byteArray out"=w1325:T1)  [unwired: 18 in]
          n399 = Bundle By Name(cluster=w1327, "Data"=w1325, "Error #"=w1328, "Data Descriptor"="C:N") -> (w1326:T2)
        }
      }
      n400 = case "Default?" shown="False" w11 {
        tunnel: w12 -> [w21 _]
        tunnel: w10 -> [w20 _]
        frame False {
          n401 = call "DeviceBase.set device state.vi"("i ref in"=w20, "implicit"=TRUE, "device error"=w21) -> ()  [unwired: 14 in, 3 out]
        }
        frame True {
        }
      }
    }
    frame Error {
    }
  }
  "answer cluster" <- w8
  "i ref out" <- w4
  "error out" <- w3
